vi "op_Pixel sweep.vi"(0 "EQ folder path Refnum":refnum<vi>, 1 "HV enable button":bool caption="High Voltage enable", 2 "HV parameters Refnum":refnum<vi>, 3 "HV level Refnum":refnum<vi>, 4 "HV string Refnum":refnum<vi>, 5 "Stop ACQ button Refnum":refnum<vi>, 6 "ACQ Parameters (cluster)":T2={"Acquisition Mode"=0, "Pulse width"=0, "DTP period"=1, "Number of events"=4000} caption="Acquisition Parameters" {"Number of events" min=1; "DTP period" min=1; "Pulse width" items=["25 ns", "50 ns", "75 ns", "100 ns"]; "Acquisition Mode" items=["Normal", "Pedestal", "Test Pulse", "Test Pulse trigger & synchronous"]}, 7 "Events to acquire Refnum":refnum<vi>, 8 "error tick Refnum":refnum<vi>, 9 "ACQ events fets Refnum":refnum<vi>, 10 "Operation text Refnum":refnum<vi>, 11 "ACQ events fets A Refnum":refnum<vi>, 12 "Busy Refnum":refnum<vi>, 13 "ACQ events fets B Refnum":refnum<vi>, 14 "Addresses Cluster":T1={"ENA1"=FALSE, "IP address 1"="172.16.14.22", "ENA2"=FALSE, "IP address 2"="172.16.14.23"}, 15 "etapa# terminals refnums":T3, 17 "GbReg params":u8[](array[numeric])=[32, 32], 19 "LayerChipIDs":u16[](array[numeric])=[65535, 65535] format="%04x", 27 "Itest parameter":cluster{"Itest tipus":bool, "I test":u8}={"Itest tipus"=TRUE, "I test"=1} caption="I test parameter" {"I test" max=63 step=1}) -> (23 "Folder path: acquisition reports":path=path "C:/VIPauto/Files/LayerID/Acquisition/yyyymmdd_hh-mm-ss_Leak#_HV#")   [LabVIEW 2015, in "VIPM2.lvlib"]
uses:
  VIPM2.lvlib
panel:
  out "Chip ID list 2":u32[](array[numeric]) format="%.0x"
  out "Layer ID list 2 (ordered)":u32[](array[numeric]) format="%.0x"
  out "All ID list 2":u32[](array[numeric]) format="%.0x"
  out "All ID list 1":u32[](array[numeric]) format="%.0x"
  out "Layer ID list 1 (ordered)":u32[](array[numeric]) format="%.0x"
  out "Chip ID list 1":u32[](array[numeric]) format="%.0x"
  # "Operation: Pixel sweep ACQuisition, with HV (refnums)"
  # "Analog Vref low"
  # "Gb THLD"
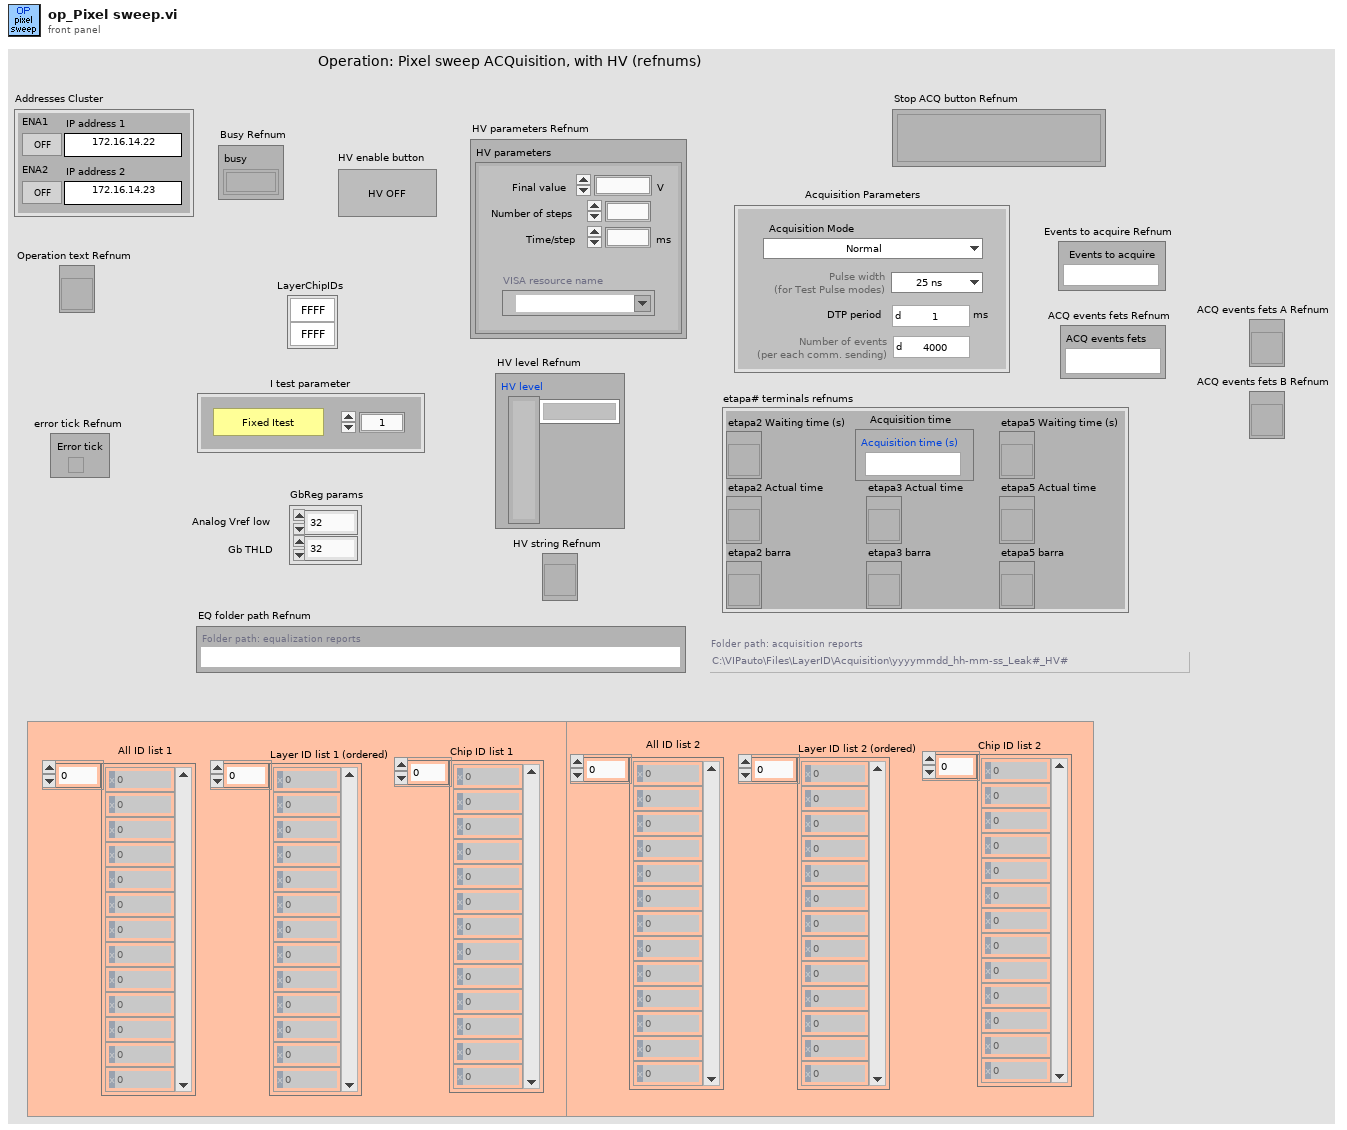
[diagram p1: front panel]
types:
  T1 = cluster{"ENA1":bool, "IP address 1":string, "ENA2":bool, "IP address 2":string}
  T2 = cluster{"Acquisition Mode":u32, "Pulse width":u32, "DTP period":u32, "Number of events":u32}
  T3 = cluster{"etapa2 Waiting time (s)":refnum<vi>, "etapa2 Actual time":refnum<vi>, "etapa2 barra":refnum<vi>, "etapa3 Actual time":refnum<vi>, "etapa3 barra":refnum<vi>, "etapa5 Waiting time (s)":refnum<vi>, "etapa5 Actual time":refnum<vi>, "etapa5 barra":refnum<vi>, "Acquisition time":refnum<vi>}
  T4 = enum8{"Enabled", "Disabled", "Disabled and Grayed Out"}
  T5 = cluster{"Final value":i16, "Number of steps":u8, "Time/step":u16, "Output Off Behavior":u16, "VISA resource name":refnum<visa-resource-name>}
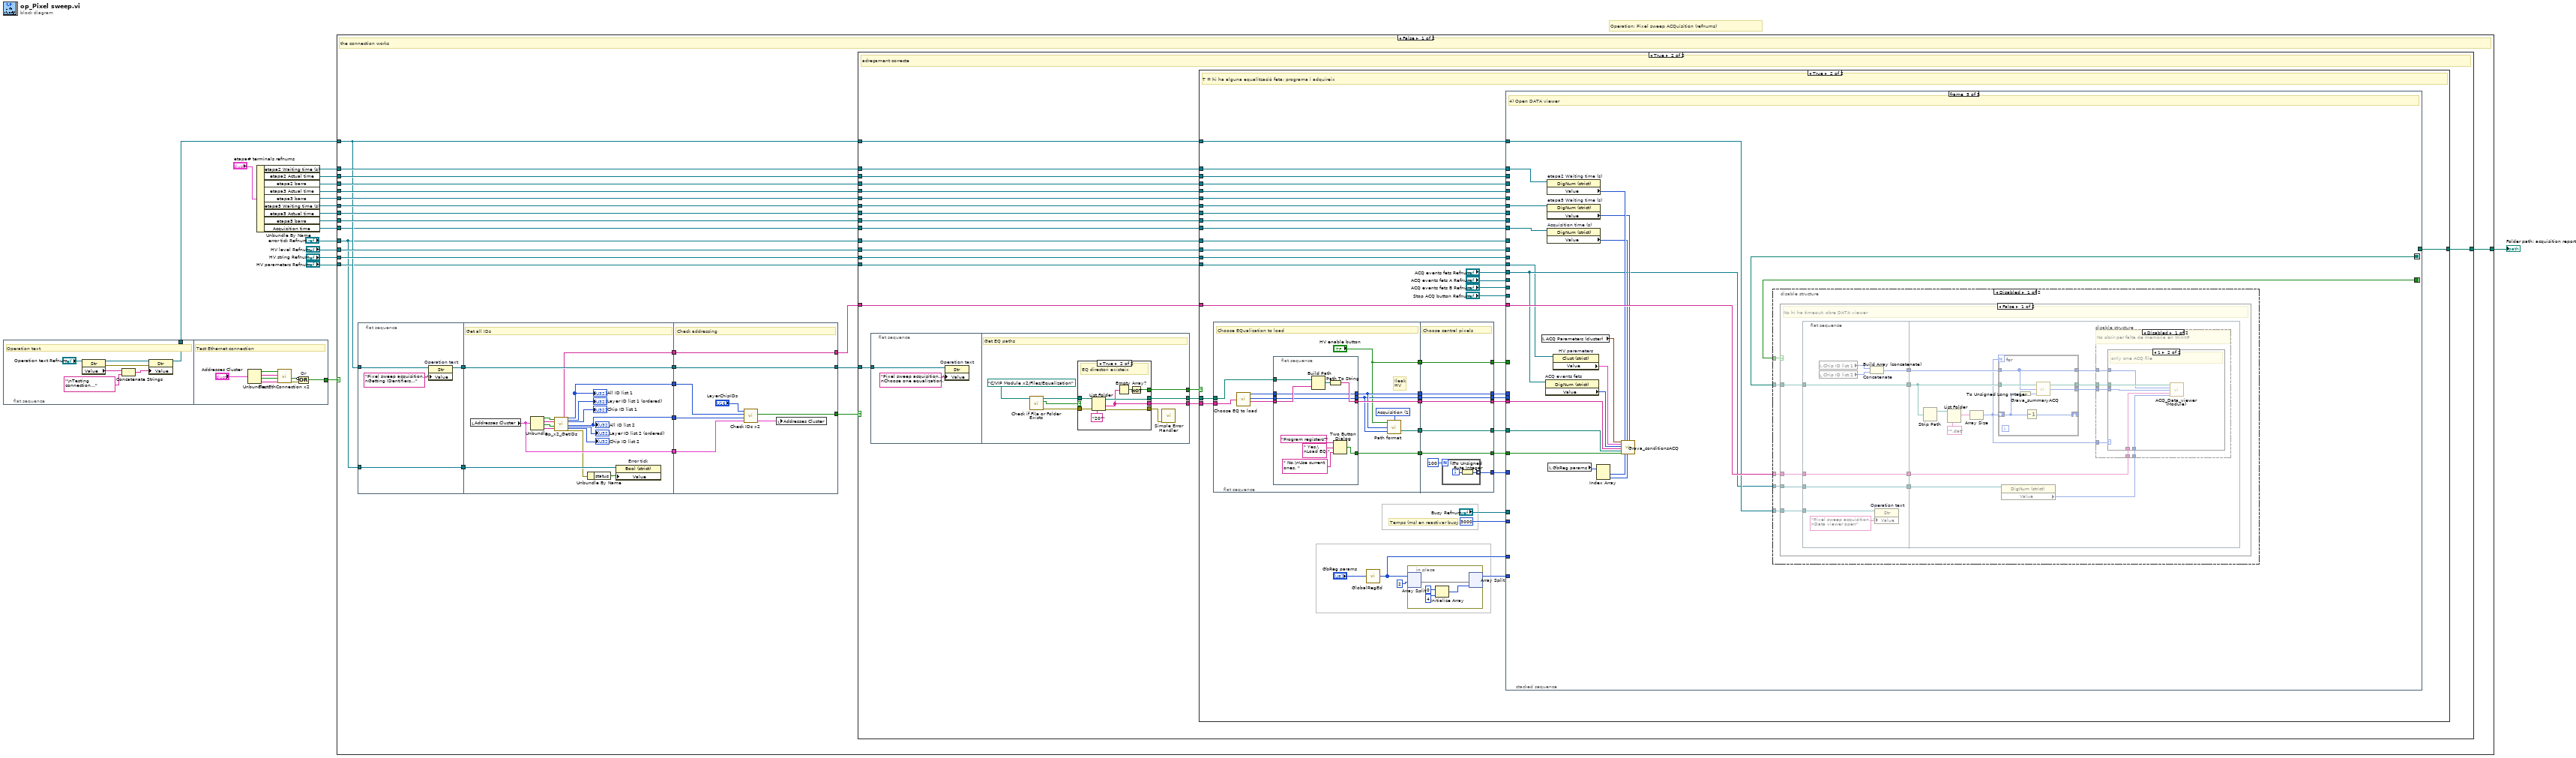
[diagram p0: block diagram]
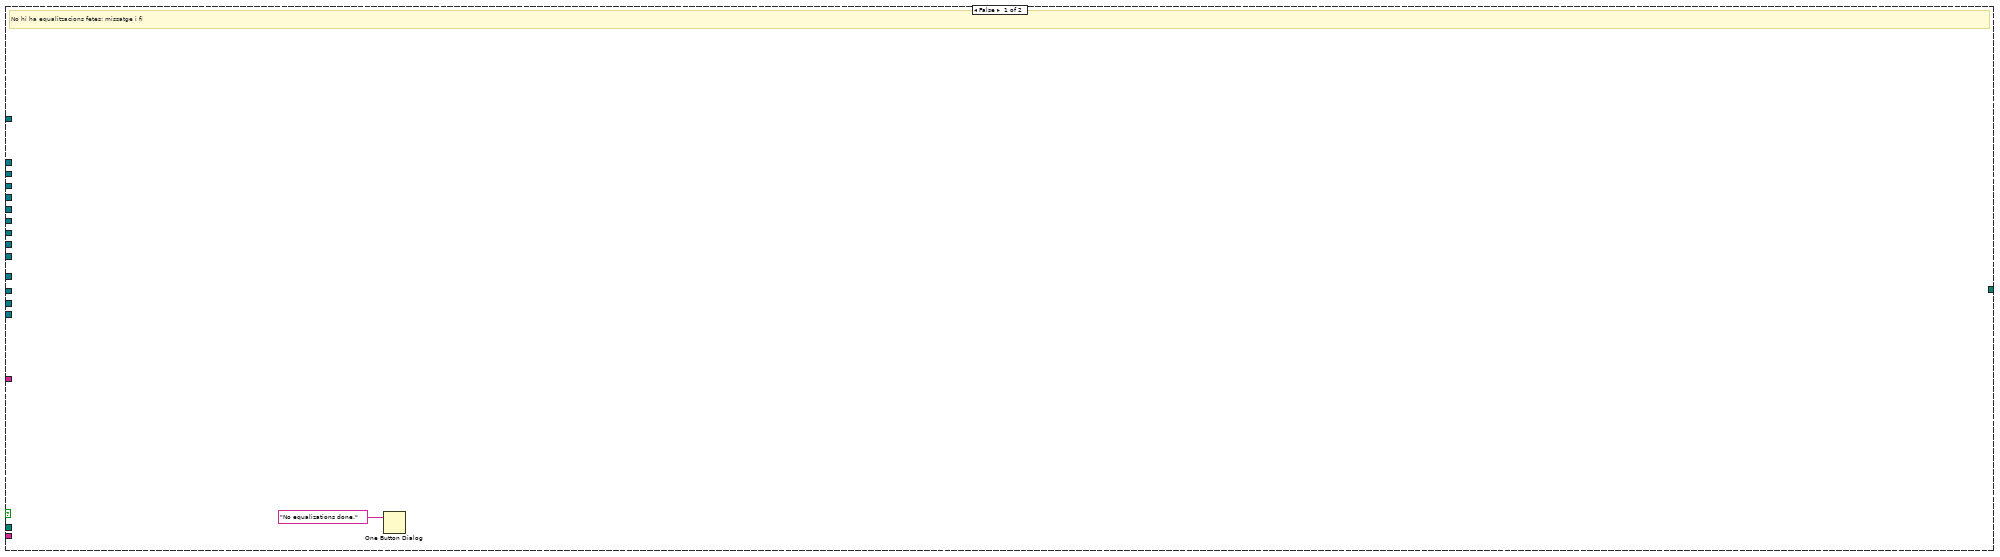
[diagram p4: hidden frame]
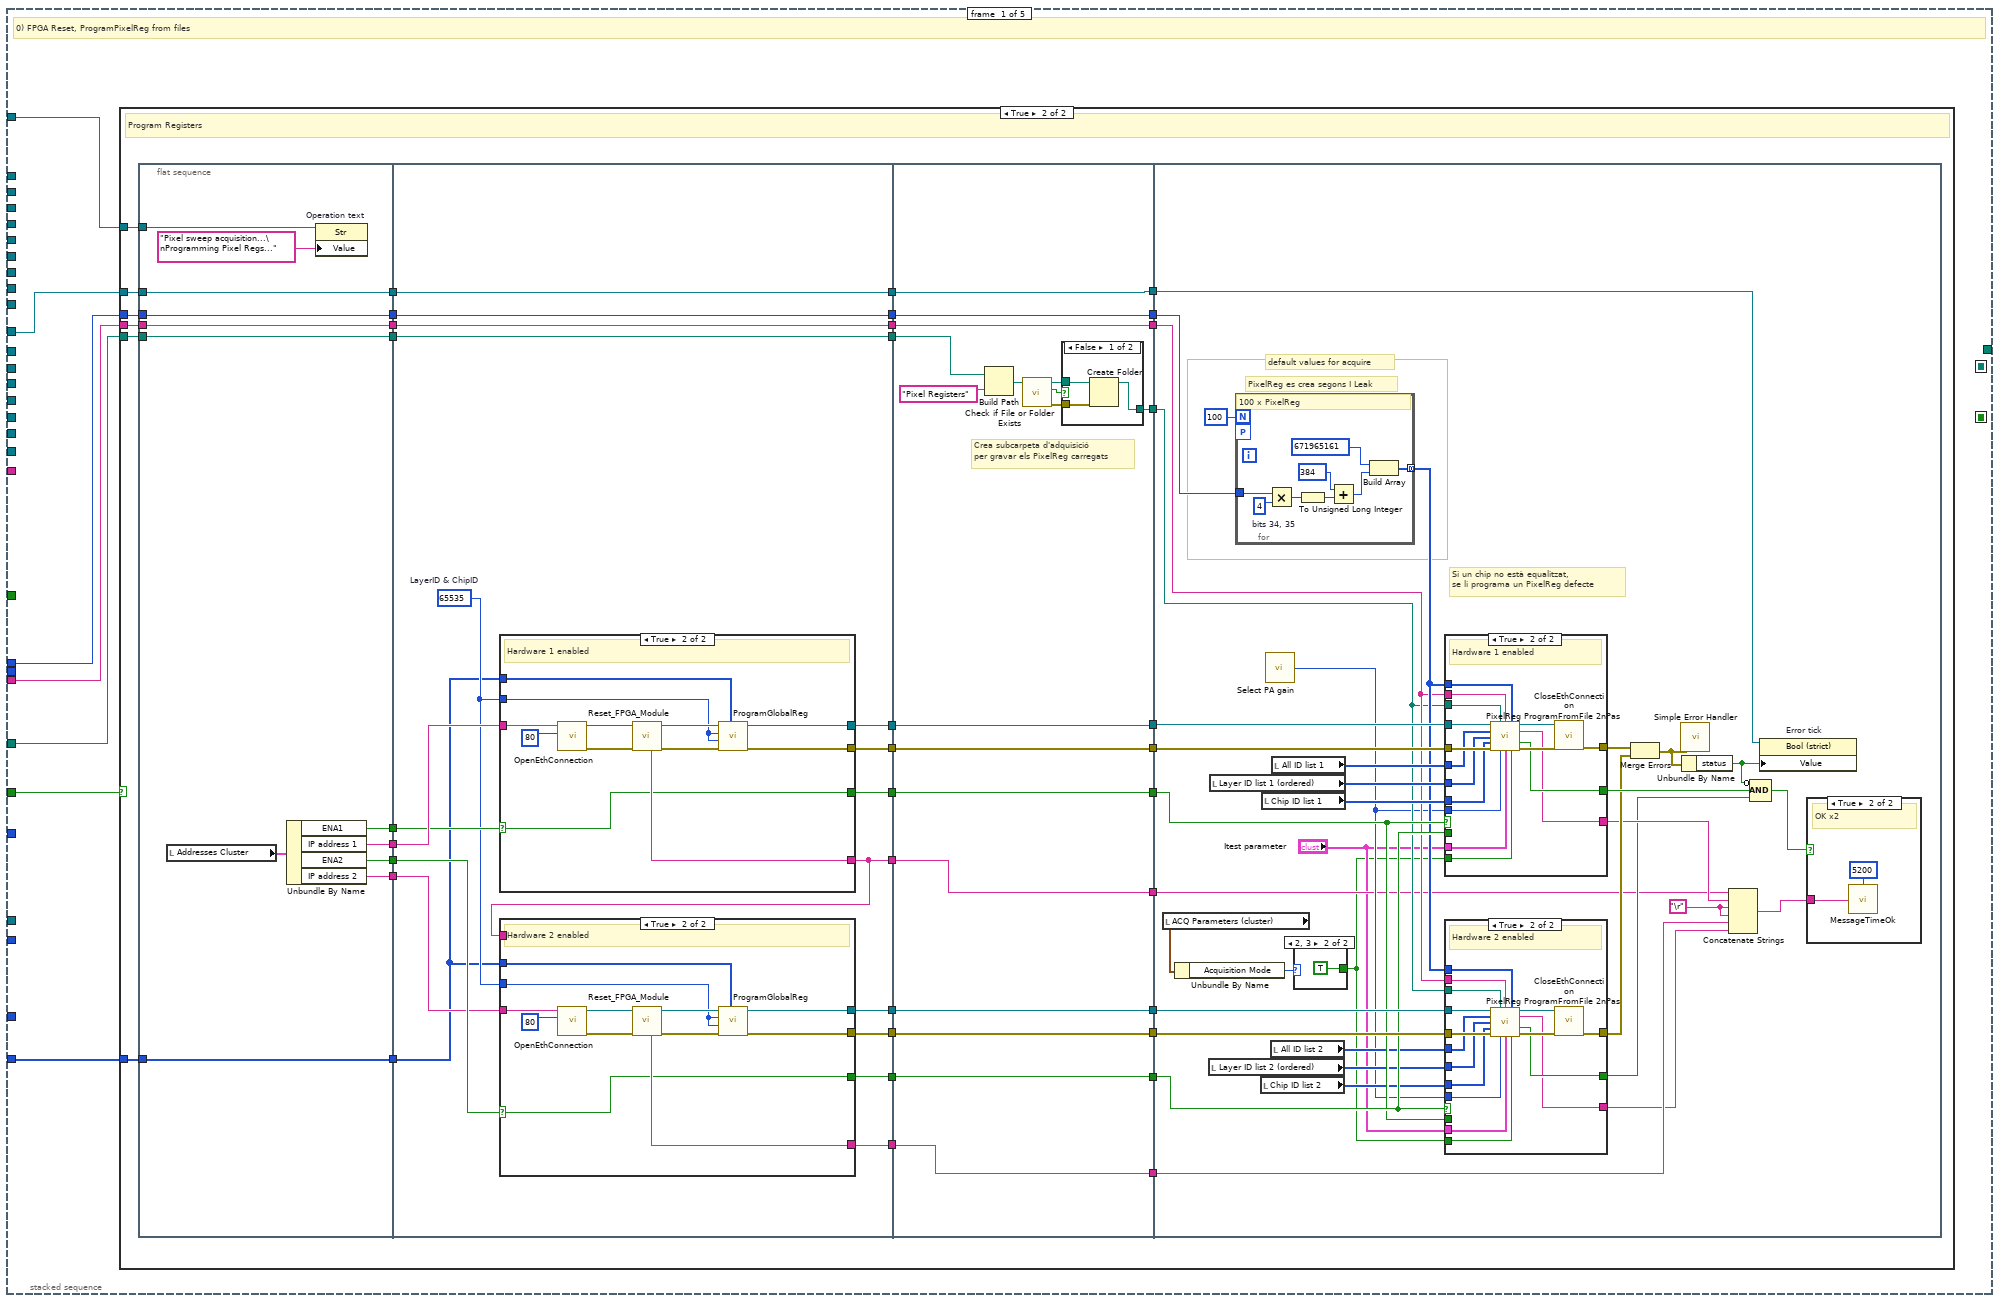
[diagram p5: hidden frame]
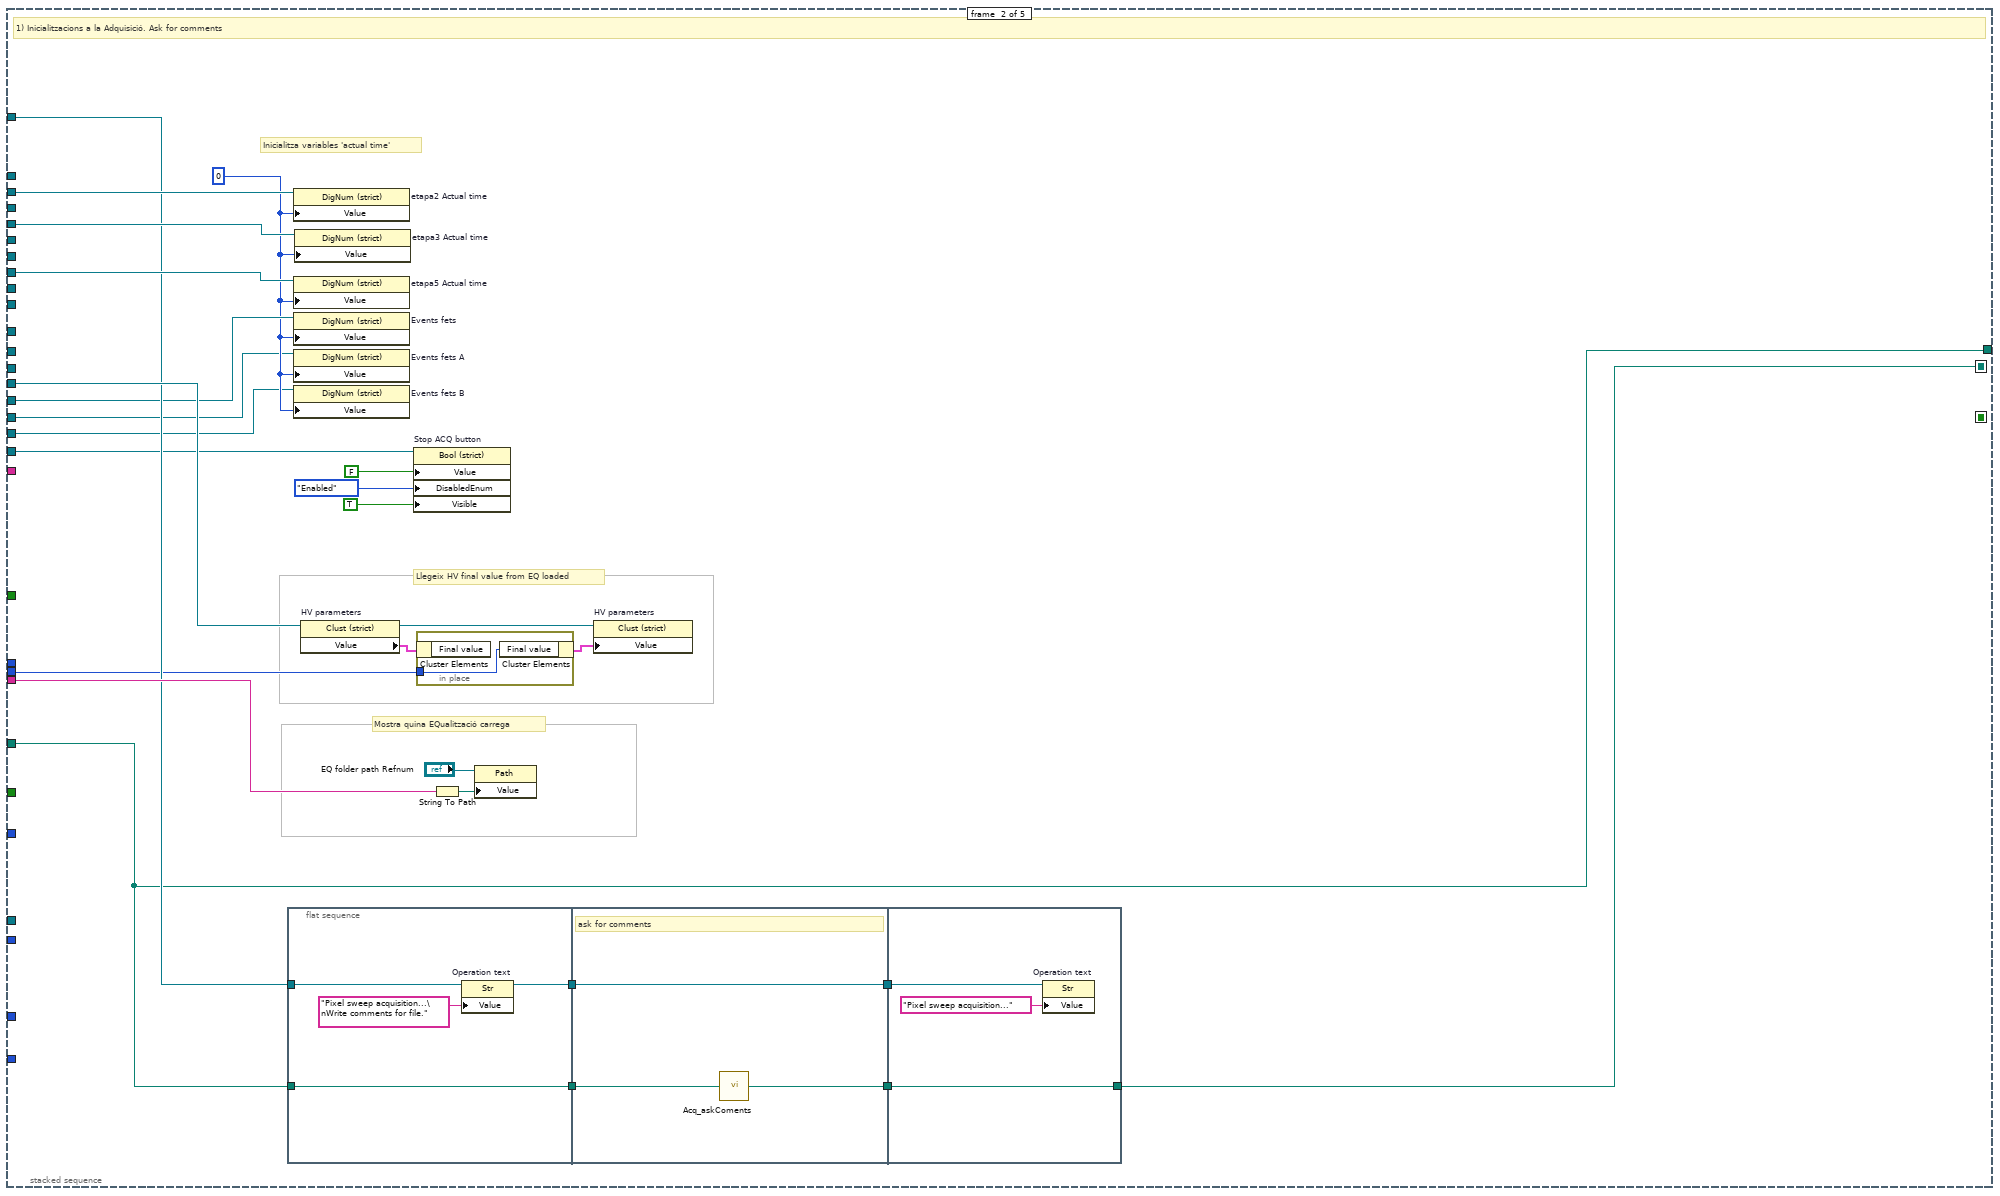
[diagram p14: hidden frame]
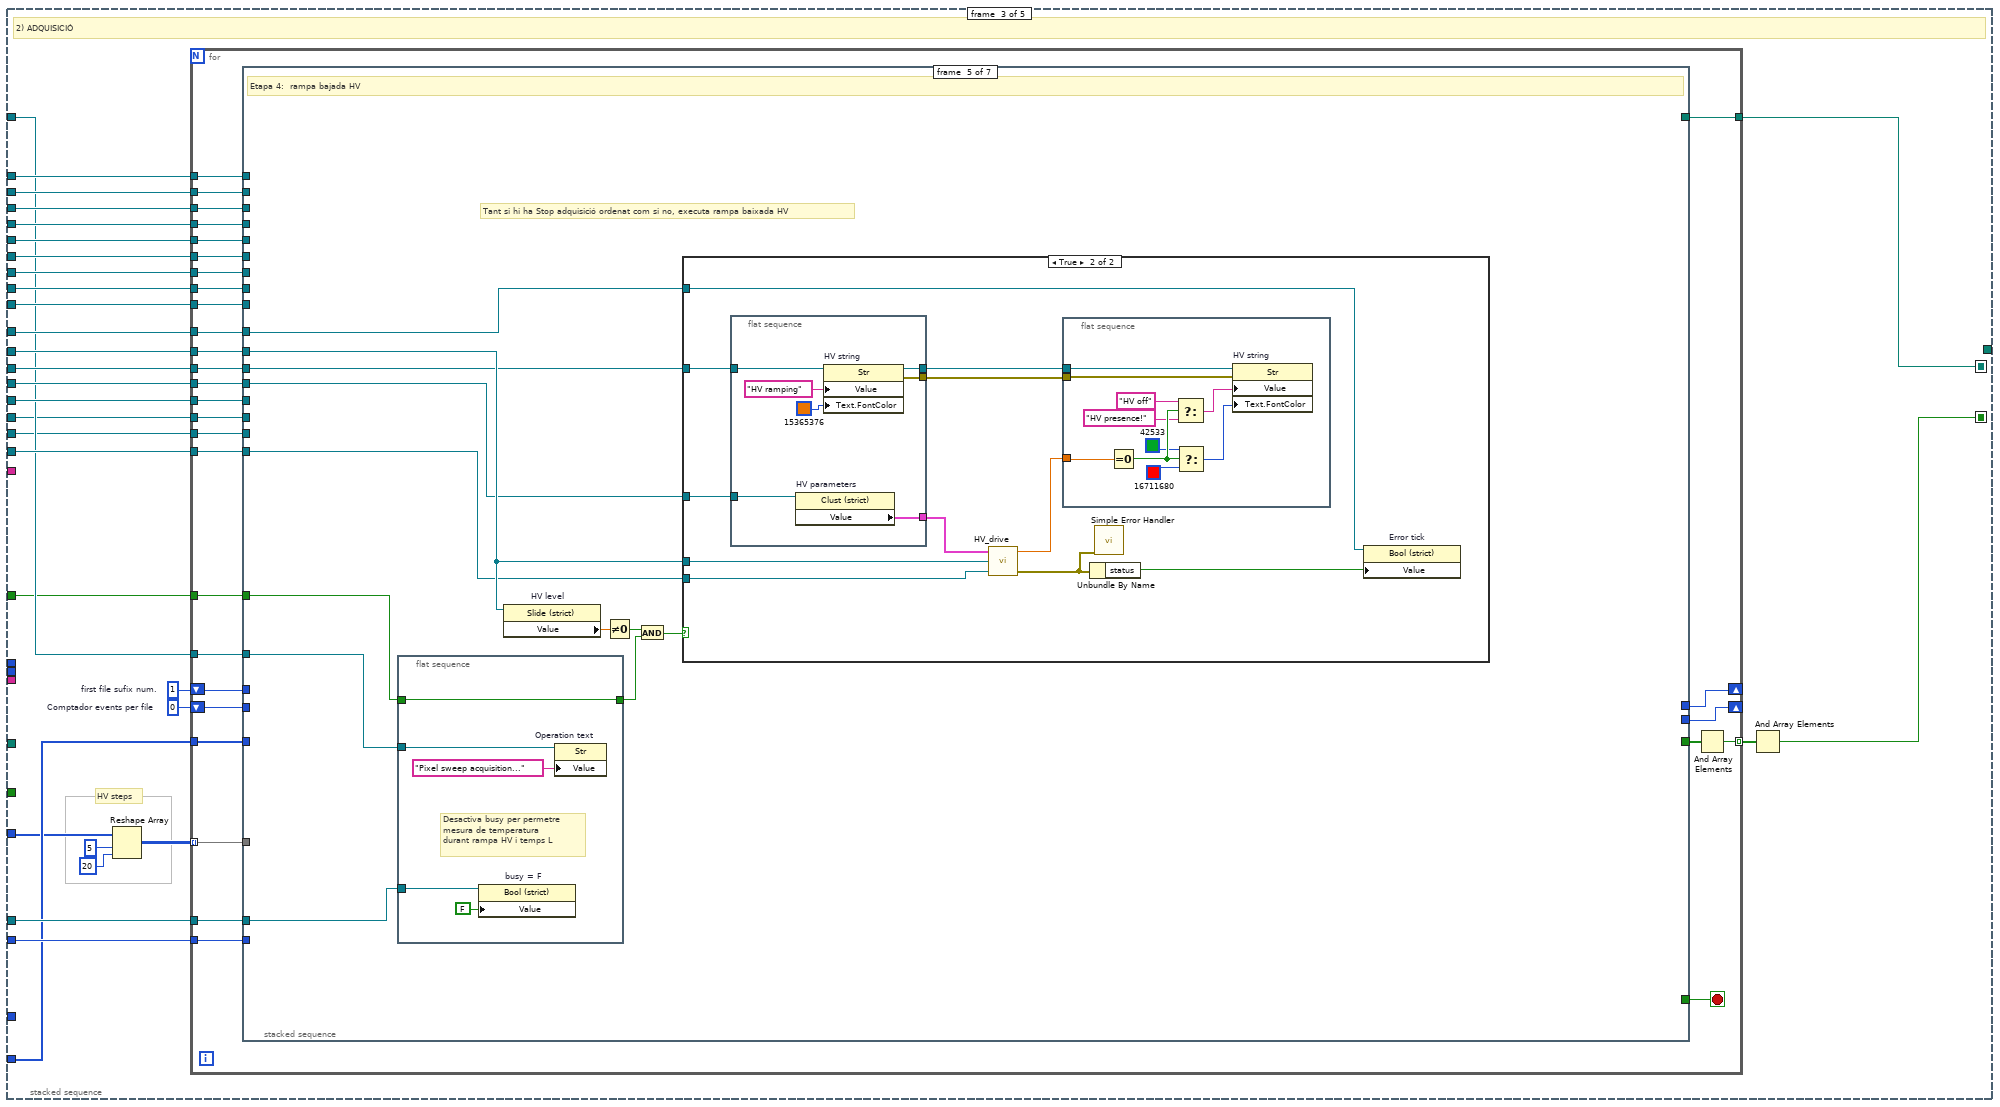
[diagram p15: hidden frame]
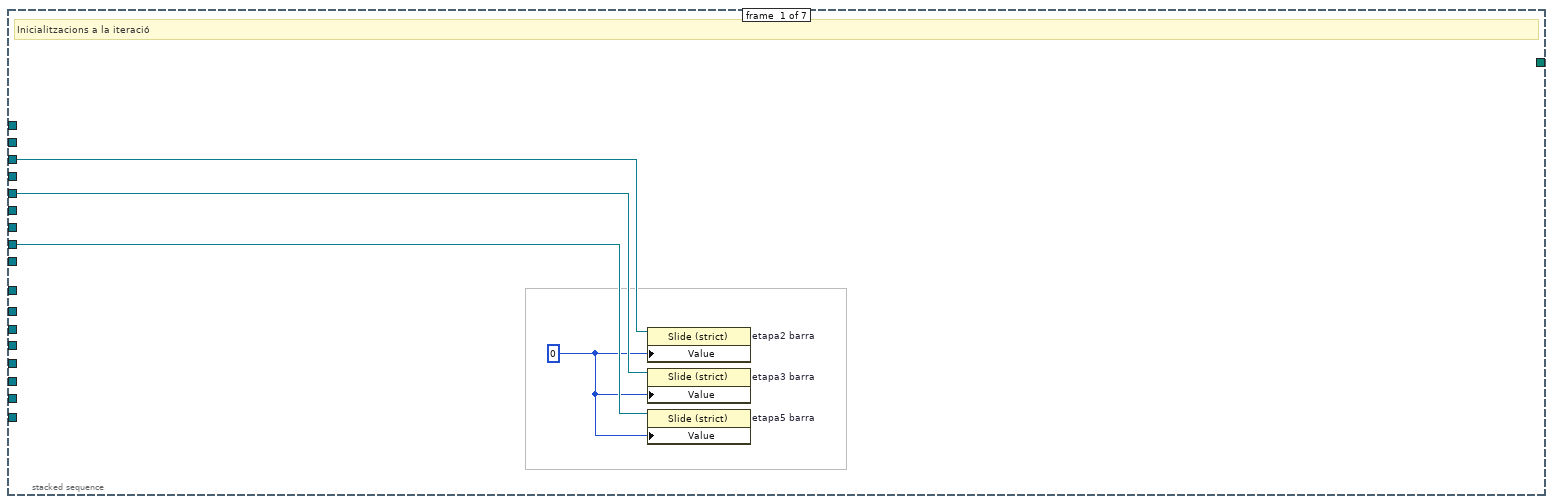
[diagram p16: hidden frame]
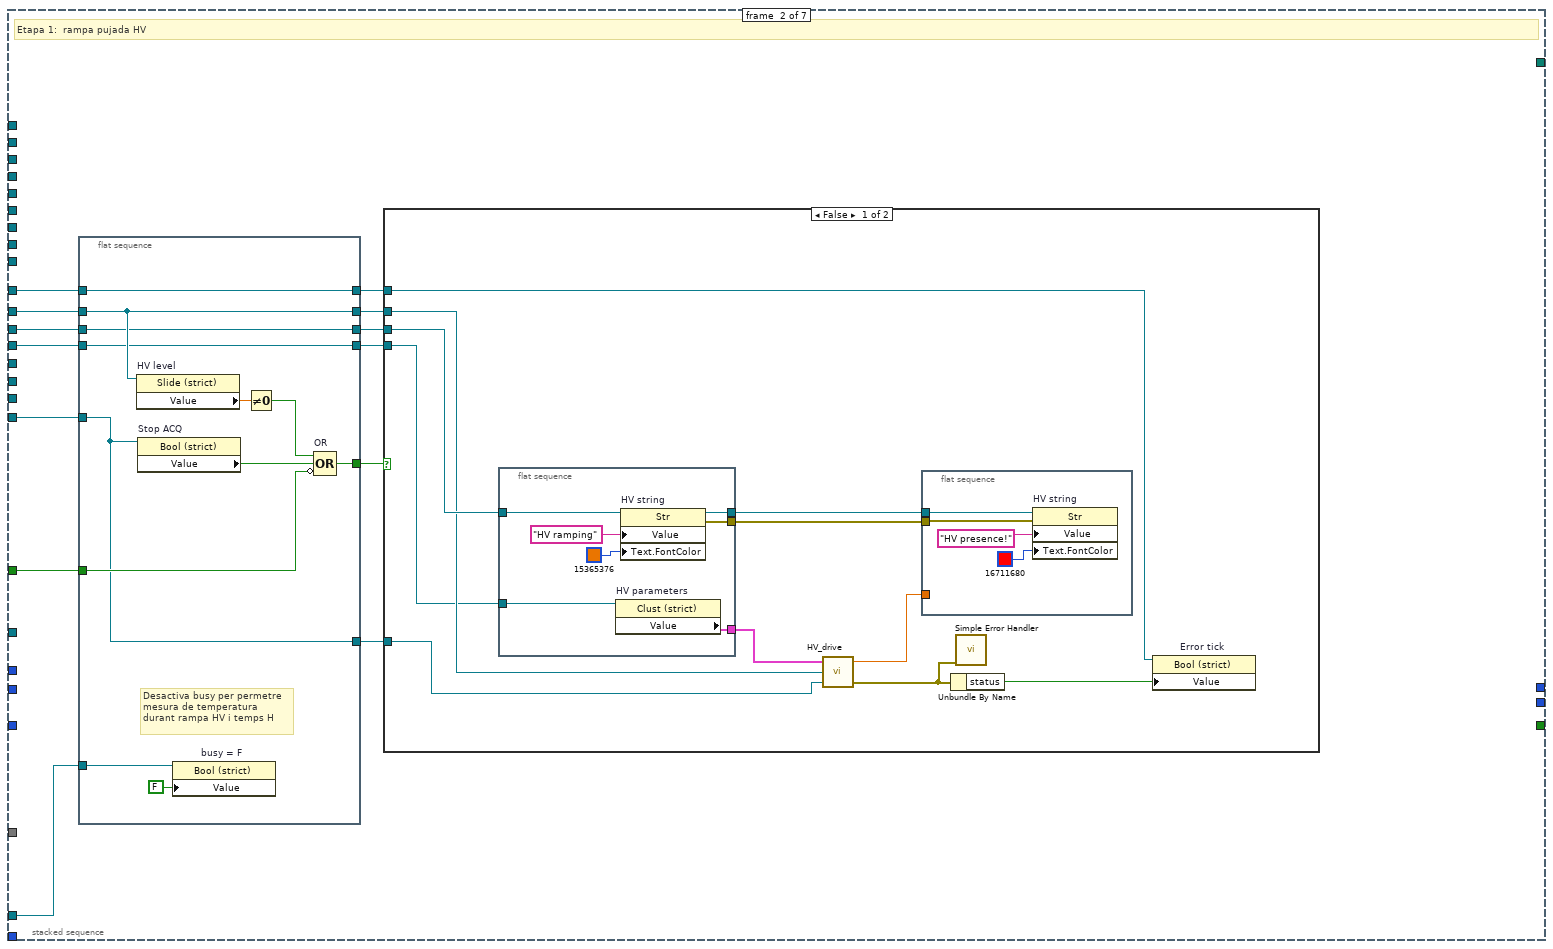
[diagram p17: hidden frame]
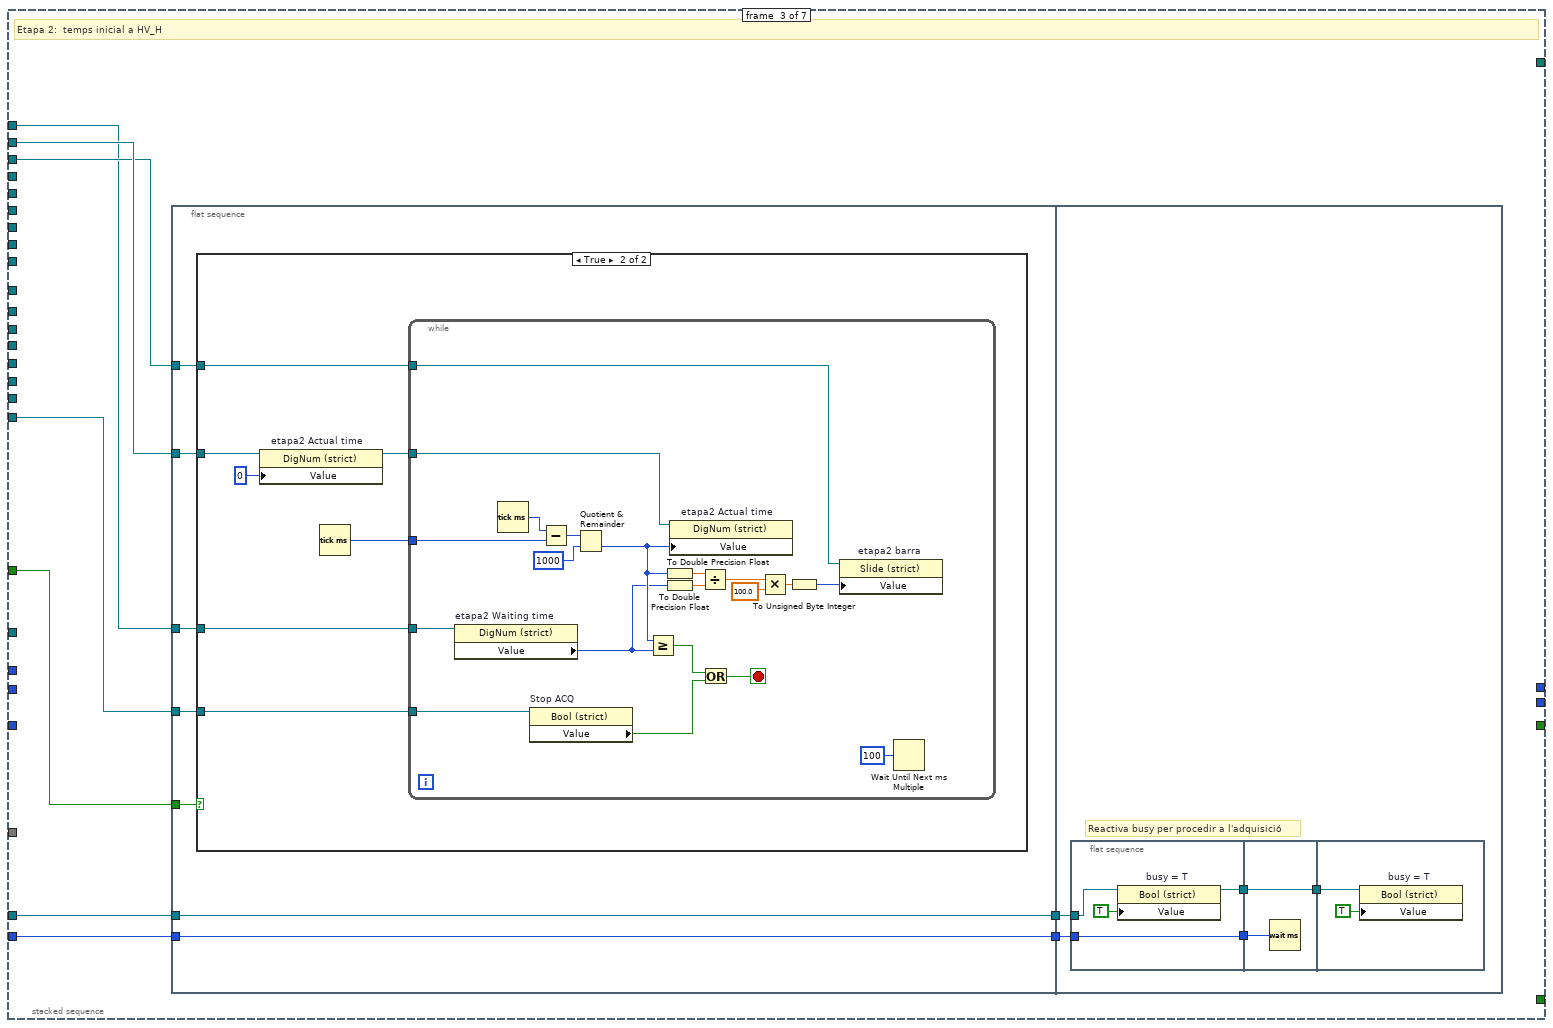
[diagram p19: hidden frame]
diagram:
  # "Operation: Pixel sweep ACQuisition (refnums)"
  n1 = flat-sequence {
    tunnel: [w18] -> w7
    tunnel: [w30] -> w17
    frame #0 {
      # "Operation text"
      n2 = property class="Str"(reference="Operation text Refnum") -> (reference out=w21:refnum<vi>, error out=w20:errorcluster, "Value"=w23:string)  [unwired: 1 in]
      n3 = Concatenate Strings "Concatenate Strings"(w23, "\nTesting connection..." ("string")) -> (w19:string)
      n4 = property class="Str"(reference=w21, error in=w20, "Value"=w19) -> (reference out=w18:refnum<vi>)  [unwired: 1 out]
    }
    frame #1 {
      # "Test Ethernet connection"
      n5 = Unbundle("Addresses Cluster") -> ("ENA1"=w28:bool, "IP address 1"=w27:string, "ENA2"=w26:bool, "IP address 2"=w25:string)
      n6 = call "TestEthConnection x2.vi"("IP address 2"=w25, "ENA2"=w26, "IP address 1"=w27, "ENA1"=w28) -> ("error out"=w31:errorcluster, "Answers OK?"=w32:bool)  [unwired: 6 in]
      n7 = Compound Arithmetic op=OR "Or"(invert w32, w31) -> (w30:bool)
    }
  }
  n8 = Unbundle By Name("etapa# terminals refnums") -> ("etapa2 Waiting time (s)"=w15:refnum<vi>, "etapa2 Actual time"=w14:refnum<vi>, "etapa2 barra"=w13:refnum<vi>, "etapa3 Actual time"=w12:refnum<vi>, "etapa3 barra"=w11:refnum<vi>, "etapa5 Waiting time (s)"=w10:refnum<vi>, "etapa5 Actual time"=w9:refnum<vi>, "etapa5 barra"=w8:refnum<vi>, "Acquisition time"=w2:refnum<vi>)
  n9 = case shown="False" w17 {
    selector: w17 -> [_ w1034]
    tunnel: w15 -> [w57 _]
    tunnel: w14 -> [w56 _]
    tunnel: w13 -> [w55 _]
    tunnel: w12 -> [w54 _]
    tunnel: w11 -> [w53 _]
    tunnel: w10 -> [w52 _]
    tunnel: w9 -> [w51 _]
    tunnel: w8 -> [w50 _]
    tunnel: w7 -> [w46 _]
    tunnel: "HV level Refnum" -> [w49 _]
    tunnel: "HV string Refnum" -> [w48 _]
    tunnel: "error tick Refnum" -> [w43 w1033]
    tunnel: [w47 _] -> w1
    tunnel: "HV parameters Refnum" -> [w45 _]
    tunnel: w2 -> [w44 _]
    frame False {
      # "the connection works"
      n10 = flat-sequence {
        tunnel: w46 -> [w61]
        tunnel: w43 -> [w58]
        tunnel: [w60] -> w42
        tunnel: [w58] -> w41
        tunnel: w42 -> [w67]
        tunnel: w41 -> [w68]
        tunnel: [w67] -> w39
        tunnel: [w66] -> w38
        tunnel: [w65] -> w36
        tunnel: [w64] -> w35
        tunnel: [w63] -> w34
        tunnel: [w84] -> w37
        tunnel: [w85] -> w40
        tunnel: w39 -> [w85]
        tunnel: w38 -> [w84]
        tunnel: w36 -> [w81]
        tunnel: w35 -> [w82]
        tunnel: w34 -> [w83]
        tunnel: [w78] -> w33
        frame #0 {
          n11 = property on="Operation text" class="Str"(reference=w61, "Value"="Pixel sweep acquisition...\nGetting IDentifiers...") -> (reference out=w60:refnum<vi>)  [unwired: 1 in, 1 out]
        }
        frame #1 {
          # "Get all IDs"
          n12 = local read "Addresses Cluster"() -> (w63:T1)
          n13 = Unbundle(w63) -> ("ENA1"=w70:bool, "IP address 1"=w71:string, "ENA2"=w73:bool, "IP address 2"=w72:string)
          n14 = call "op_x2_GetIDs.vi"("ENA1"=w70, "IP address 1"=w71, "ENA2"=w73, "IP address 2"=w72) -> ("summary IDs"=w66:string, "All ID list 1"=w65:u32[], "Layer ID list 1 (ordered)"=→"Layer ID list 1 (ordered)":u32[], "Chip ID list 1"=→"Chip ID list 1":u32[], "All ID list 2"=w64:u32[], "Layer ID list 2 (ordered)"=→"Layer ID list 2 (ordered)":u32[], "Chip ID list 2"=→"Chip ID list 2":u32[], "error out"=w62:errorcluster)  [unwired: 16 in]
          "All ID list 1" <- w65
          "All ID list 2" <- w64
          n15 = Unbundle By Name(w62) -> ("status"=w69:bool)
          n16 = property on="Error tick" class="Bool (strict)"(reference=w68, "Value"=w69) -> ()  [unwired: 1 in, 2 out]
        }
        frame #2 {
          # "Check addressing"
          n17 = call "Check IDs x2.vi"("Addresses Cluster in"=w83, "All ID list 2"=w82, "All ID list 1"=w81, "LayerChipIDs"="LayerChipIDs") -> ("Addresses Cluster out"=w79:T1, "OK?"=w78:bool)  [unwired: 6 in]
          n18 = local write "Addresses Cluster"(w79) -> ()
        }
      }
      n19 = case shown="True" w33 {
        tunnel: w57 -> [_ w105]
        tunnel: w56 -> [_ w104]
        tunnel: w55 -> [_ w103]
        tunnel: w54 -> [_ w102]
        tunnel: w53 -> [_ w101]
        tunnel: w52 -> [_ w100]
        tunnel: w51 -> [_ w99]
        tunnel: w50 -> [_ w98]
        tunnel: w49 -> [_ w97]
        tunnel: w48 -> [_ w96]
        tunnel: [_ w95] -> w47
        tunnel: w46 -> [_ w94]
        tunnel: w45 -> [_ w90]
        tunnel: w44 -> [_ w89]
        tunnel: w43 -> [_ w88]
        tunnel: w40 -> [_ w87]
        tunnel: w37 -> [_ w86]
        frame False {
          # "adreçament incorrecte"
        }
        frame True {
          # "adreçament correcte"
          n20 = flat-sequence {
            tunnel: w87 -> [w106]
            tunnel: [w115] -> w93
            tunnel: [w114] -> w92
            tunnel: [w113] -> w91
            frame #0 {
              n21 = property on="Operation text" class="Str"(reference=w106, "Value"="Pixel sweep acquisition...\nChoose one equalization.") -> ()  [unwired: 1 in, 2 out]
            }
            frame #1 {
              # "Get EQ paths"
              n22 = call <vilib>:"Check if File or Folder Exists.vi"("path"=path "C:/VIP Module x2/Files/Equalization") -> ("error out"=w109:errorcluster, "file or folder exists?"=w110:bool, "dup path"=w111:path)  [unwired: 8 in]
              n23 = case shown="True" w110 {
                selector: w110 -> [w118 _]
                tunnel: w111 -> [w117 w124]
                tunnel: w109 -> [w116 w123]
                tunnel: [w118 w120] -> w115
                tunnel: [w117 w121] -> w114
                tunnel: [w116 w122] -> w108
                tunnel: [_ w119] -> w113
                frame False {
                  # "no EQs"
                }
                frame True {
                  # "EQ directori existeix"
                  n24 = List Folder(path=w124, pattern="20*", error in=w123) -> (path out=w121:path, folder names=w119:string[], error out=w122:errorcluster)  [unwired: 1 in, 1 out]
                  n25 = Empty Array?(array=w119) -> (empty?=w125:bool)
                  n26 = Not(x=w125) -> (.not. x?=w120:bool)
                }
              }
              n27 = call <vilib>:"Simple Error Handler.vi"("error in (no error)"=w108) -> ()  [unwired: 4 in, 5 out]
            }
          }
          n28 = case shown="True" w93 {
            tunnel: w105 -> [_ w168]
            tunnel: w104 -> [_ w167]
            tunnel: w103 -> [_ w166]
            tunnel: w102 -> [_ w165]
            tunnel: w101 -> [_ w164]
            tunnel: w100 -> [_ w163]
            tunnel: w99 -> [_ w162]
            tunnel: w98 -> [_ w161]
            tunnel: w97 -> [_ w160]
            tunnel: w96 -> [_ w159]
            tunnel: [_ w158] -> w95
            tunnel: w94 -> [_ w157]
            tunnel: w88 -> [_ w156]
            tunnel: w92 -> [_ w155]
            tunnel: w91 -> [_ w154]
            tunnel: w90 -> [_ w150]
            tunnel: w89 -> [_ w147]
            tunnel: w86 -> [_ w145]
            frame False {
              # "No hi ha equalitzacions fetes: missatge i fi"
              n29 = One Button Dialog(message="No equalizations done.") -> ()  [unwired: 1 in, 1 out]
            }
            frame True {
              # "Temps (ms) en reactivar busy"
              # "T = hi ha alguna equalització feta: programa i adquireix"
              n30 = flat-sequence {
                tunnel: w155 -> [w181]
                tunnel: w154 -> [w182]
                tunnel: [w179] -> w140
                tunnel: [w174] -> w139
                tunnel: [w177] -> w138
                tunnel: [w183] -> w137
                tunnel: [w178] -> w136
                tunnel: ["HV enable button"] -> w135
                tunnel: [w197] -> w141
                tunnel: [w198] -> w144
                tunnel: [w199] -> w149
                tunnel: [w200] -> w151
                tunnel: [w201] -> w152
                tunnel: [w202] -> w153
                tunnel: w140 -> [w202]
                tunnel: w139 -> [w201]
                tunnel: w138 -> [w200]
                tunnel: w137 -> [w199]
                tunnel: w136 -> [w198]
                tunnel: w135 -> [w197]
                tunnel: [w195] -> w134
                frame #0 {
                  w184 = u8 1 items=["Equalization", "Acquisition"] ("Operation type")
                  # "Ileak\nHV"
                  # "Choose EQualization to load"
                  n31 = call "Choose EQ to load.vi"("EQ folders"=w182) -> ("I Leakage"=w176:u8, "HV last value"=w175:i16, "loaded EQ folder"=w180:string)  [unwired: 5 in]
                  n32 = flat-sequence {
                    tunnel: w181 -> [w194]
                    tunnel: w180 -> [w193]
                    tunnel: [w191] -> w179
                    tunnel: [w190] -> w178
                    tunnel: [w186] -> w177
                    tunnel: w176 -> [w186]
                    tunnel: w175 -> [w185]
                    tunnel: [w185] -> w174
                    frame #0 {
                      n33 = Build Path(base path=w194, name or relative path=w193) -> (appended path=w192:path)
                      n34 = Path To String(path=w192) -> (string=w191:string)
                      n35 = Two Button Dialog(message="Program registers?", 1:" No.\nUse current ones. " ("F button name (\"Cancel\")"), 2:" Yes.\nLoad EQ." ("T button name (\"OK\")")) -> (T button?=w190:bool)
                    }
                  }
                  n36 = call "Path format.vi"("Operation type"=w184, "HV level"=w174, "I leakage"=w177, "HV enable button"="HV enable button") -> ("folder path"=w183:path)  [unwired: 1 in]
                }
                frame #1 {
                  # "Choose central pixels"
                  n37 = for {
                    N: 100 -> [_]
                    tunnel: [w203] -> w195 mode=indexing
                    i -> [w204]
                    n38 = To Unsigned Byte Integer(number=w204) -> (unsigned 8bit integer=w203:u8)
                  }
                }
              }
              n39 = call "GlobalRegEd.vi"("params"="GbReg params") -> ("Global Reg out"=w129:u32[])  [unwired: 4 in]
              n40 = in-place {
                n41 = in-place-split #1(w129, 2) -> (w172:u32[])  [unwired: 1 out]
                n42 = Initialize Array "Initialize Array"(u32 0, 4 ("dimension size")) -> (w169:u32[])
                n43 = in-place-split #1(w172, w169) -> (w130:u32[])  [unwired: 1 out]
              }
              n44 = stacked-sequence {
                seq-local: [_ _ w449 _ _] -> [_ _ _ _ w979]
                seq-local: [_ w422 _ _ _] -> [_ _ w465 _ w978]
                tunnel: w157 -> [w211 w427 w461 w899 w976]
                tunnel: w168 -> [_ _ w479 _ w959]
                tunnel: w167 -> [_ w437 w478 _ _]
                tunnel: w166 -> [_ _ w477 _ _]
                tunnel: w165 -> [_ w436 w476 _ _]
                tunnel: w164 -> [_ _ w475 _ _]
                tunnel: w163 -> [_ _ w474 _ w960]
                tunnel: w162 -> [_ w435 w473 _ _]
                tunnel: w161 -> [_ _ w472 _ _]
                tunnel: w156 -> [w210 _ w469 w901 _]
                tunnel: w160 -> [_ _ w471 _ _]
                tunnel: w159 -> [_ _ w470 _ _]
                tunnel: [_ w420 _ _ _] -> w158
                tunnel: w153 -> [w209 w428 _ _ w964]
                tunnel: w152 -> [_ w426 _ _ _]
                tunnel: w151 -> [w208 _ _ _ _]
                tunnel: w150 -> [_ w434 w468 _ w962]
                tunnel: w149 -> [w207 w420 _ _ w965]
                tunnel: "Stop ACQ button Refnum" -> [_ w419 w467 w898 _]
                tunnel: w147 -> [_ _ w466 _ w961]
                tunnel: "ACQ events fets Refnum" -> [_ w415 w464 _ w963]
                tunnel: w145 -> [_ _ _ _ w977]
                tunnel: w144 -> [w206 _ _ _ w966]
                tunnel: "Busy Refnum" -> [_ _ w463 w897 _]
                tunnel: u32 3000 -> [_ _ w462 _ _]
                tunnel: w141 -> [_ _ w460 _ _]
                tunnel: w134 -> [_ _ w454 _ _]
                tunnel: "ACQ events fets A Refnum" -> [_ w413 w459 _ _]
                tunnel: "ACQ events fets B Refnum" -> [_ w412 w458 _ _]
                tunnel: w130 -> [w205 _ w455 _ _]
                tunnel: w129 -> [_ _ _ w896 _]
                frame #0 {
                  # "0) FPGA Reset, ProgramPixelReg from files"
                  n45 = case shown="True" w206 {
                    tunnel: w211 -> [_ w237]
                    tunnel: w210 -> [_ w236]
                    tunnel: w209 -> [_ w235]
                    tunnel: w208 -> [_ w234]
                    tunnel: w207 -> [_ w233]
                    tunnel: w205 -> [_ w213]
                    frame False {
                      # "Use current registers values"
                    }
                    frame True {
                      # "Program Registers"
                      n46 = flat-sequence {
                        tunnel: w237 -> [w261]
                        tunnel: [w260] -> w250
                        tunnel: w236 -> [w260]
                        tunnel: [w259] -> w249
                        tunnel: w235 -> [w259]
                        tunnel: [w258] -> w248
                        tunnel: w234 -> [w258]
                        tunnel: [w257] -> w247
                        tunnel: w233 -> [w257]
                        tunnel: [w255] -> w232
                        tunnel: [w254] -> w231
                        tunnel: [w253] -> w230
                        tunnel: [w252] -> w229
                        tunnel: w213 -> [w251]
                        tunnel: [w251] -> w212
                        tunnel: [w280] -> w246
                        tunnel: w250 -> [w280]
                        tunnel: w249 -> [w279]
                        tunnel: [w279] -> w245
                        tunnel: w248 -> [w278]
                        tunnel: [w278] -> w244
                        tunnel: w247 -> [w277]
                        tunnel: [w277] -> w243
                        tunnel: w232 -> [w272]
                        tunnel: w231 -> [w267]
                        tunnel: w230 -> [w273]
                        tunnel: w229 -> [w266]
                        tunnel: [w276] -> w228
                        tunnel: [w275] -> w227
                        tunnel: [w274] -> w226
                        tunnel: [w263] -> w225
                        tunnel: [w271] -> w224
                        tunnel: [w270] -> w223
                        tunnel: [w269] -> w222
                        tunnel: [w268] -> w221
                        tunnel: w212 -> [w264]
                        tunnel: [w314] -> w242
                        tunnel: [w313] -> w241
                        tunnel: [w324] -> w240
                        tunnel: w246 -> [w324]
                        tunnel: [w323] -> w239
                        tunnel: w245 -> [w323]
                        tunnel: [w322] -> w238
                        tunnel: w244 -> [w322]
                        tunnel: w243 -> [w316]
                        tunnel: w228 -> [w314]
                        tunnel: w227 -> [w313]
                        tunnel: w226 -> [w312]
                        tunnel: w225 -> [w308]
                        tunnel: w224 -> [w311]
                        tunnel: w223 -> [w310]
                        tunnel: w222 -> [w309]
                        tunnel: w221 -> [w307]
                        tunnel: [w315] -> w220
                        tunnel: [w312] -> w219
                        tunnel: [w311] -> w218
                        tunnel: [w310] -> w217
                        tunnel: [w309] -> w216
                        tunnel: [w308] -> w215
                        tunnel: [w307] -> w214
                        tunnel: w242 -> [w359]
                        tunnel: w241 -> [w358]
                        tunnel: w240 -> [w361]
                        tunnel: w239 -> [w341]
                        tunnel: w238 -> [w356]
                        tunnel: w220 -> [w340]
                        tunnel: w219 -> [w349]
                        tunnel: w218 -> [w352]
                        tunnel: w217 -> [w351]
                        tunnel: w216 -> [w350]
                        tunnel: w215 -> [w334]
                        tunnel: w214 -> [w337]
                        frame #0 {
                          n47 = local read "Addresses Cluster"() -> (w256:T1)
                          n48 = Unbundle By Name(w256) -> ("ENA1"=w255:bool, "IP address 1"=w253:string, "ENA2"=w254:bool, "IP address 2"=w252:string)
                          n49 = property on="Operation text" class="Str"(reference=w261, "Value"="Pixel sweep acquisition...\nProgramming Pixel Regs...") -> ()  [unwired: 1 in, 2 out]
                        }
                        frame #1 {
                          w265 = u32 65535  # LayerID & ChipID
                          n50 = case shown="True" w272 {
                            selector: w272 -> [w294 w295]
                            tunnel: w265 -> [_ w297]
                            tunnel: [_ w301] -> w276
                            tunnel: [_ w300] -> w275
                            tunnel: [_ w299] -> w263
                            tunnel: w264 -> [_ w298]
                            tunnel: w273 -> [_ w296]
                            tunnel: [w294 w295] -> w274
                            frame False {
                              # "Hardware 1 not enabled"
                            }
                            frame True {
                              # "Hardware 1 enabled"
                              n51 = call "OpenEthConnection.vi"("Port"=u16 80, "IP address"=w296) -> ("error out"=w305:errorcluster, "connection ID out"=w306:refnum<k5>)  [unwired: 7 in, 1 out]
                              n52 = call "Reset_FPGA_Module.vi"("error in (no error)"=w305, "connection ID"=w306) -> ("error out"=w302:errorcluster, "connection ID out"=w303:refnum<k5>, "Answer to Reset"=w299:string)  [unwired: 7 in]
                              n53 = call "ProgramGlobalReg.vi"("Global Reg"=w298, "error in (no error)"=w302, "ChipID"=w297, "LayerID"=w297, "connection ID"=w303) -> ("error out"=w300:errorcluster, "connection ID out"=w301:refnum<k5>)  [unwired: 2 in, 3 out]
                            }
                          }
                          n54 = case shown="True" w267 {
                            selector: w267 -> [w281 w282]
                            tunnel: w265 -> [_ w284]
                            tunnel: [_ w288] -> w271
                            tunnel: [_ w287] -> w270
                            tunnel: [_ w286] -> w268
                            tunnel: w264 -> [_ w285]
                            tunnel: w266 -> [_ w283]
                            tunnel: [w281 w282] -> w269
                            tunnel: w263 -> [_ _]
                            frame False {
                              # "Hardware 2 not enabled"
                            }
                            frame True {
                              # "Hardware 2 enabled"
                              n55 = call "OpenEthConnection.vi"("Port"=u16 80, "IP address"=w283) -> ("error out"=w292:errorcluster, "connection ID out"=w293:refnum<k5>)  [unwired: 7 in, 1 out]
                              n56 = call "Reset_FPGA_Module.vi"("error in (no error)"=w292, "connection ID"=w293) -> ("error out"=w289:errorcluster, "connection ID out"=w290:refnum<k5>, "Answer to Reset"=w286:string)  [unwired: 7 in]
                              n57 = call "ProgramGlobalReg.vi"("Global Reg"=w285, "error in (no error)"=w289, "ChipID"=w284, "LayerID"=w284, "connection ID"=w290) -> ("error out"=w287:errorcluster, "connection ID out"=w288:refnum<k5>)  [unwired: 2 in, 3 out]
                            }
                          }
                        }
                        frame #2 {
                          # "Crea subcarpeta d'adquisició\nper gravar els PixelReg carregats"
                          n58 = Build Path(base path=w316, name or relative path="Pixel Registers") -> (appended path=w320:path)
                          n59 = call <vilib>:"Check if File or Folder Exists.vi"("path"=w320) -> ("error out"=w317:errorcluster, "file or folder exists?"=w319:bool, "dup path"=w318:path)  [unwired: 8 in]
                          n60 = case shown="False" w319 {
                            tunnel: w318 -> [w327 w328]
                            tunnel: w317 -> [w326 _]
                            tunnel: [w325 w328] -> w315
                            frame False {
                              n61 = Create Folder(path (use dialog)=w327, error in=w326) -> (created path=w325:path)  [unwired: 1 in, 2 out]
                            }
                            frame True {
                            }
                          }
                        }
                        frame #3 {
                          w338 = "\r"
                          # "Si un chip no està equalitzat,\nse li programa un PixelReg defecte"
                          # "default values for acquire"
                          # "PixelReg es crea segons I Leak"
                          n62 = local read "ACQ Parameters (cluster)"() -> (w331:T2)
                          n63 = Unbundle By Name(w331) -> ("Acquisition Mode"=w330:u32)
                          n64 = local read "Layer ID list 2 (ordered)"() -> (w347:u32[])
                          n65 = local read "Layer ID list 1 (ordered)"() -> (w354:u32[])
                          n66 = for {
                            N: 100 -> [_]
                            tunnel: w356 -> [w405]
                            tunnel: [w402] -> w342 mode=concatenating
                            workers-P: _ -> [_]
                            w409 = u8 4  # bits 34, 35
                            # "100 x PixelReg"
                            n67 = Multiply(x=w405, y=w409) -> (x*y=w407:u8)
                            n68 = To Unsigned Long Integer(number=w407) -> (unsigned 32bit integer=w406:u32)
                            n69 = Add(x=u32 384, y=w406) -> (x+y=w403:u32)
                            n70 = Build Array(u32 671965161 ("Numeric"), w403) -> (w402:u32[])
                          }
                          n71 = local read "Chip ID list 2"() -> (w346:u32[])
                          n72 = local read "Chip ID list 1"() -> (w353:u32[])
                          n73 = call "Select PA gain.vi"() -> ("PA gain selected"=w336:u8)  [unwired: 5 in]
                          n74 = local read "All ID list 2"() -> (w348:u32[])
                          n75 = local read "All ID list 1"() -> (w355:u32[])
                          n76 = case shown="2, 3" w330 {
                            tunnel: [_ TRUE] -> w329
                            frame Default {
                            }
                            frame 2, 3 {
                            }
                          }
                          n77 = case shown="True" w349 {
                            tunnel: [w385 w401] -> w344
                            tunnel: w359 -> [_ w400]
                            tunnel: w358 -> [w385 w399]
                            tunnel: [w384 w396] -> w357
                            tunnel: w342 -> [_ w395]
                            tunnel: w341 -> [_ w394]
                            tunnel: w340 -> [_ w393]
                            tunnel: [_ w392] -> w339
                            tunnel: w355 -> [_ w389]
                            tunnel: w354 -> [_ w390]
                            tunnel: w353 -> [_ w391]
                            tunnel: w350 -> [w384 _]
                            tunnel: w336 -> [_ w388]
                            tunnel: "Itest parameter" -> [_ w387]
                            tunnel: w329 -> [_ w386]
                            frame False {
                              # "Hardware 1 not enabled"
                            }
                            frame True {
                              # "Hardware 1 enabled"
                              n78 = call "PixelReg ProgramFromFile 2nPas.vi"("connection ID"=w400, "ACQ PxReg folder"=w393, "EQ folder path"=w394, "PixelReg (hex)"=w395, "All ID list"=w389, "Layer ID list"=w390, "Chip ID list"=w391, "error in (no error)"=w399, "PA gain"=w388, "Itest parameter"=w387, "TP EN"=w386) -> ("connection ID out"=w398:refnum<k5>, "done message"=w392:string, "All checks OK"=w396:bool, "error out (no error)"=w397:errorcluster)  [unwired: 1 out]
                              n79 = call "CloseEthConnection.vi"("error in (no error)"=w397, "connection ID"=w398) -> ("error out"=w401:errorcluster)  [unwired: 9 in]
                            }
                          }
                          n80 = case shown="True" w350 {
                            tunnel: [w367 w383] -> w343
                            tunnel: w352 -> [_ w382]
                            tunnel: w351 -> [w367 w381]
                            tunnel: [w366 w378] -> w335
                            tunnel: w342 -> [_ w377]
                            tunnel: w341 -> [_ w376]
                            tunnel: w340 -> [_ w375]
                            tunnel: [_ w374] -> w333
                            tunnel: w348 -> [_ w371]
                            tunnel: w347 -> [_ w372]
                            tunnel: w346 -> [_ w373]
                            tunnel: w349 -> [w366 _]
                            tunnel: w336 -> [_ w370]
                            tunnel: "Itest parameter" -> [_ w369]
                            tunnel: w329 -> [_ w368]
                            frame False {
                              # "Hardware 2 not enabled"
                            }
                            frame True {
                              # "Hardware 2 enabled"
                              n81 = call "PixelReg ProgramFromFile 2nPas.vi"("connection ID"=w382, "ACQ PxReg folder"=w375, "EQ folder path"=w376, "PixelReg (hex)"=w377, "All ID list"=w371, "Layer ID list"=w372, "Chip ID list"=w373, "error in (no error)"=w381, "PA gain"=w370, "Itest parameter"=w369, "TP EN"=w368) -> ("connection ID out"=w380:refnum<k5>, "done message"=w374:string, "All checks OK"=w378:bool, "error out (no error)"=w379:errorcluster)  [unwired: 1 out]
                              n82 = call "CloseEthConnection.vi"("error in (no error)"=w379, "connection ID"=w380) -> ("error out"=w383:errorcluster)  [unwired: 9 in]
                            }
                          }
                          n83 = Merge Errors(w344, w343) -> (w345:errorcluster)
                          n84 = call <vilib>:"Simple Error Handler.vi"("error in (no error)"=w345) -> ()  [unwired: 4 in, 5 out]
                          n85 = Unbundle By Name(w345) -> ("status"=w360:bool)
                          n86 = Concatenate Strings "Concatenate Strings"(w334, w339, w338, w338, w337, w333) -> (w363:string)
                          n87 = Compound Arithmetic op=AND(invert w360, w357, w335) -> (w362:bool)
                          n88 = property on="Error tick" class="Bool (strict)"(reference=w361, "Value"=w360) -> ()  [unwired: 1 in, 2 out]
                          n89 = case shown="True" w362 {
                            tunnel: w363 -> [_ w411]
                            frame False {
                              # "error"
                            }
                            frame True {
                              # "OK x2"
                              n90 = call "MessageTimeOk.vi"("time (ms)"=5200, "missage"=w411) -> ()  [unwired: 4 in]
                            }
                          }
                        }
                      }
                    }
                  }
                }
                frame #1 {
                  w414 = u32 0 ("Value")
                  # "Mostra quina EQualització carrega"
                  # "Llegeix HV final value from EQ loaded"
                  # "Inicialitza variables 'actual time'"
                  # "1) Inicialitzacions a la Adquisició. Ask for comments"
                  n91 = flat-sequence {
                    tunnel: w427 -> [w440]
                    tunnel: [w439] -> w423
                    tunnel: [w438] -> w421
                    tunnel: w420 -> [w438]
                    tunnel: [w444] -> w425
                    tunnel: [w443] -> w424
                    tunnel: w423 -> [w443]
                    tunnel: w421 -> [w442]
                    tunnel: [w447] -> w422
                    tunnel: w425 -> [w447]
                    tunnel: w424 -> [w446]
                    frame #0 {
                      n92 = property on="Operation text" class="Str"(reference=w440, "Value"="Pixel sweep acquisition...\nWrite comments for file.") -> (reference out=w439:refnum<vi>)  [unwired: 1 in, 1 out]
                    }
                    frame #1 {
                      # "ask for comments"
                      n93 = call "Acq_askComents.vi"("Folder path"=w442) -> ("Complete file path"=w444:path)  [unwired: 4 in]
                    }
                    frame #2 {
                      n94 = property on="Operation text" class="Str"(reference=w446, "Value"="Pixel sweep acquisition...") -> ()  [unwired: 1 in, 2 out]
                    }
                  }
                  n95 = property on="etapa2 Actual time" class="DigNum (strict)"(reference=w437, "Value"=w414) -> ()  [unwired: 1 in, 2 out]
                  n96 = property on="etapa5 Actual time" class="DigNum (strict)"(reference=w435, "Value"=w414) -> ()  [unwired: 1 in, 2 out]
                  n97 = property on="Events fets" class="DigNum (strict)"(reference=w415, "Value"=w414) -> ()  [unwired: 1 in, 2 out]
                  n98 = property on="Events fets A" class="DigNum (strict)"(reference=w413, "Value"=w414) -> ()  [unwired: 1 in, 2 out]
                  n99 = property on="Events fets B" class="DigNum (strict)"(reference=w412, "Value"=w414) -> ()  [unwired: 1 in, 2 out]
                  n100 = property on="etapa3 Actual time" class="DigNum (strict)"(reference=w436, "Value"=w414) -> ()  [unwired: 1 in, 2 out]
                  n101 = property on="HV parameters" class="Clust (strict)"(reference=w434) -> (reference out=w431:refnum<vi>, "Value"=w433:T5)  [unwired: 1 in, 1 out]
                  n102 = property on="Stop ACQ button" class="Bool (strict)"(reference=w419, "Value"=FALSE, "DisabledEnum"=T4."Enabled" ("Disabled"), "Visible"=TRUE) -> ()  [unwired: 1 in, 2 out]
                  n103 = in-place {
                    in-place-border: w426 -> [w448]
                    n104 = in-place-cluster #2(w433) -> ()  [unwired: 1 out]
                    n105 = in-place-cluster #2("Final value"=w448) -> (w432:T5)
                  }
                  n106 = String To Path(string=w428) -> (path=w429:path)
                  n107 = property class="Path"(reference="EQ folder path Refnum", "Value"=w429) -> ()  [unwired: 1 in, 2 out]
                  n108 = property on="HV parameters" class="Clust (strict)"(reference=w431, "Value"=w432) -> ()  [unwired: 1 in, 2 out]
                }
                frame #2 {
                  w456 = u32 0  # Comptador events per file
                  w457 = u32 1  # first file sufix num.
                  # "HV steps"
                  # "2) ADQUISICIÓ"
                  n109 = Reshape Array "Reshape Array"(w454, 5 ("dimension size"), 20 ("dimension size")) -> (w451:u8[][])
                  n110 = for {
                    tunnel: w479 -> [w510]
                    tunnel: w478 -> [w509]
                    tunnel: w477 -> [w508]
                    tunnel: w476 -> [w507]
                    tunnel: w475 -> [w506]
                    tunnel: w474 -> [w505]
                    tunnel: w473 -> [w504]
                    tunnel: w472 -> [w503]
                    tunnel: w471 -> [w502]
                    tunnel: w470 -> [w501]
                    tunnel: w469 -> [w500]
                    tunnel: w468 -> [w499]
                    tunnel: w467 -> [w498]
                    tunnel: w460 -> [w497]
                    tunnel: w466 -> [w496]
                    tunnel: w465 -> [w495]
                    tunnel: [w482] -> w450 mode=indexing
                    tunnel: w464 -> [w494]
                    tunnel: w463 -> [w493]
                    tunnel: w462 -> [w492]
                    tunnel: w461 -> [w491]
                    tunnel: w459 -> [w490]
                    tunnel: w458 -> [w489]
                    shift-right: [w480] -> _
                    shift-left: w457 -> [w488]
                    shift-right: [w481] -> _
                    shift-left: w456 -> [w487]
                    tunnel: w455 -> [w486]
                    tunnel: w451 -> [w485] mode=indexing
                    stop <- w484 stop-if-true
                    n111 = stacked-sequence {
                      tunnel: w510 -> [_ _ w568 _ _ _ _]
                      tunnel: w509 -> [_ _ w570 _ _ _ _]
                      tunnel: w508 -> [w514 _ w569 _ _ _ _]
                      tunnel: w507 -> [_ _ _ w631 _ _ _]
                      tunnel: w506 -> [w513 _ _ w630 _ _ _]
                      tunnel: w505 -> [_ _ _ _ _ w848 _]
                      tunnel: w504 -> [_ _ _ _ _ w849 _]
                      tunnel: w503 -> [w512 _ _ _ _ w847 _]
                      tunnel: w502 -> [_ w526 _ _ w806 _ _]
                      tunnel: w501 -> [_ w519 _ _ w805 _ _]
                      tunnel: w500 -> [_ w522 _ w633 w804 _ _]
                      tunnel: w499 -> [_ w517 _ _ w803 _ _]
                      tunnel: w498 -> [_ w527 w567 w627 w798 w846 w892]
                      tunnel: w497 -> [_ w524 w566 _ w800 w845 _]
                      tunnel: w496 -> [_ _ _ w635 _ _ _]
                      tunnel: w495 -> [_ _ _ w634 _ _ _]
                      tunnel: [_ _ _ w632 _ _ _] -> w483
                      tunnel: [_ _ _ _ _ _ w891] -> w484
                      tunnel: w494 -> [_ _ _ w628 _ _ _]
                      tunnel: w493 -> [_ w516 w564 _ w799 w843 _]
                      tunnel: w492 -> [_ _ w562 _ _ w841 _]
                      tunnel: w491 -> [_ _ _ w626 w796 _ _]
                      tunnel: w485 -> [_ _ _ w625 _ _ _]
                      tunnel: w490 -> [_ _ _ w623 _ _ _]
                      tunnel: w489 -> [_ _ _ w624 _ _ _]
                      tunnel: w488 -> [_ _ _ w620 _ _ _]
                      tunnel: w487 -> [_ _ _ w621 _ _ _]
                      tunnel: w486 -> [_ _ _ w622 _ _ _]
                      tunnel: [_ _ _ w619 _ _ _] -> w481
                      tunnel: [_ _ _ w618 _ _ _] -> w480
                      frame #0 {
                        w511 = u8 0 ("ACQ-e2 barra")
                        # "Inicialitzacions a la iteració"
                        n112 = property on="etapa2 barra" class="Slide (strict)"(reference=w514, "Value"=w511) -> ()  [unwired: 1 in, 2 out]
                        n113 = property on="etapa3 barra" class="Slide (strict)"(reference=w513, "Value"=w511) -> ()  [unwired: 1 in, 2 out]
                        n114 = property on="etapa5 barra" class="Slide (strict)"(reference=w512, "Value"=w511) -> ()  [unwired: 1 in, 2 out]
                      }
                      frame #1 {
                        # "Etapa 1:  rampa pujada HV"
                        n115 = flat-sequence {
                          tunnel: w527 -> [w528]
                          tunnel: w526 -> [w533]
                          tunnel: [w536] -> w525
                          tunnel: w524 -> [w535]
                          tunnel: [w534] -> w523
                          tunnel: w522 -> [w534]
                          tunnel: [w533] -> w521
                          tunnel: [w532] -> w520
                          tunnel: w519 -> [w532]
                          tunnel: [w531] -> w518
                          tunnel: w517 -> [w531]
                          tunnel: w516 -> [w529]
                          tunnel: [w528] -> w515
                          frame #0 {
                            # "Desactiva busy per permetre\nmesura de temperatura\ndurant rampa HV i temps H"
                            n116 = property on="HV level" class="Slide (strict)"(reference=w533) -> ("Value"=w539:dbl)  [unwired: 1 in, 2 out]
                            n117 = property on="Stop ACQ" class="Bool (strict)"(reference=w528) -> ("Value"=w537:bool)  [unwired: 1 in, 2 out]
                            n118 = property on="busy = F" class="Bool (strict)"(reference=w529, "Value"=FALSE) -> ()  [unwired: 1 in, 2 out]
                            n119 = Not Equal To 0?(x=w539) -> (x != 0?=w538:bool)
                            n120 = Compound Arithmetic op=OR "OR"(w538, w537, invert w535) -> (w536:bool)
                          }
                        }
                        n121 = case shown="False" w525 {
                          tunnel: w520 -> [w547 _]
                          tunnel: w521 -> [w544 _]
                          tunnel: w523 -> [w543 _]
                          tunnel: w518 -> [w541 _]
                          tunnel: w515 -> [w540 _]
                          frame False {
                            n122 = flat-sequence {
                              tunnel: [w556] -> w550
                              tunnel: w547 -> [w561]
                              tunnel: [w559] -> w546
                              tunnel: [w558] -> w545
                              tunnel: w541 -> [w555]
                              frame #0 {
                                n123 = property on="HV parameters" class="Clust (strict)"(reference=w555) -> ("Value"=w556:T5)  [unwired: 1 in, 2 out]
                                n124 = property on="HV string" class="Str"(reference=w561, "Value"="HV ramping" ("HV String"), "Text.FontColor"=u32 15365376) -> (reference out=w559:refnum<vi>, error out=w558:errorcluster)  [unwired: 1 in]
                              }
                            }
                            n125 = call "HV_drive.vi"("Stop subVI Refnum"=w540, "HV level Refnum"=w544, "HV parameters"=w550) -> ("error out"=w549:errorcluster, "HV level (last value)"=w548:dbl)  [unwired: 1 in]
                            n126 = flat-sequence {
                              tunnel: w548 -> [_]
                              tunnel: w546 -> [w553]
                              tunnel: w545 -> [w552]
                              frame #0 {
                                n127 = property on="HV string" class="Str"(reference=w553, error in=w552, "Value"="HV presence!" ("HV String"), "Text.FontColor"=u32 16711680) -> ()  [unwired: 2 out]
                              }
                            }
                            n128 = Unbundle By Name(w549) -> ("status"=w542:bool)
                            n129 = call <vilib>:"Simple Error Handler.vi"("error in (no error)"=w549) -> ()  [unwired: 4 in, 5 out]
                            n130 = property on="Error tick" class="Bool (strict)"(reference=w543, "Value"=w542) -> ()  [unwired: 1 in, 2 out]
                          }
                          frame True {
                            # "executant aturada\no hi ha HV manual\no HV not enabled"
                          }
                        }
                      }
                      frame #2 {
                        # "Etapa 2:  temps inicial a HV_H"
                        n131 = flat-sequence {
                          tunnel: w570 -> [w577]
                          tunnel: w569 -> [w576]
                          tunnel: w568 -> [w575]
                          tunnel: w567 -> [w574]
                          tunnel: w566 -> [w573]
                          tunnel: [w572] -> w565
                          tunnel: w564 -> [w572]
                          tunnel: [w571] -> w563
                          tunnel: w562 -> [w571]
                          tunnel: w565 -> [w608]
                          tunnel: w563 -> [w607]
                          frame #0 {
                            n132 = case shown="True" w573 {
                              tunnel: w577 -> [_ w583]
                              tunnel: w576 -> [_ w581]
                              tunnel: w575 -> [_ w580]
                              tunnel: w574 -> [_ w579]
                              frame False {
                              }
                              frame True {
                                n133 = property on="etapa2 Actual time" class="DigNum (strict)"(reference=w583, "Value"=u32 0 ("ACQ-e2 Actual time")) -> (reference out=w582:refnum<vi>)  [unwired: 1 in, 1 out]
                                n134 = Tick Count (ms)() -> (millisecond timer value=w584:u32)
                                n135 = while {
                                tunnel: w584 -> [w603]
                                tunnel: w582 -> [w593]
                                tunnel: w580 -> [w592]
                                tunnel: w581 -> [w590]
                                tunnel: w579 -> [w586]
                                stop <- w588 stop-if-true
                                n136 = property on="etapa2 Waiting time" class="DigNum (strict)"(reference=w592) -> ("Value"=w591:u32)  [unwired: 1 in, 2 out]
                                n137 = Tick Count (ms)() -> (millisecond timer value=w604:u32)
                                n138 = property on="Stop ACQ" class="Bool (strict)"(reference=w586) -> ("Value"=w585:bool)  [unwired: 1 in, 2 out]
                                n139 = Subtract(x=w604, y=w603) -> (x-y=w602:u32)
                                n140 = Quotient & Remainder(x=w602, y=u32 1000) -> (floor(x/y)=w594:u32)  [unwired: 1 out]
                                n141 = Greater Or Equal?(x=w594, y=w591) -> (x >= y?=w587:bool)
                                n142 = To Double Precision Float(number=w594) -> (double precision float=w595:dbl)
                                n143 = To Double Precision Float(number=w591) -> (double precision float=w596:dbl)
                                n144 = property on="etapa2 Actual time" class="DigNum (strict)"(reference=w593, "Value"=w594) -> ()  [unwired: 1 in, 2 out]
                                n145 = Divide(x=w595, y=w596) -> (x/y=w599:dbl)
                                n146 = Or(x=w587, y=w585) -> (x .or. y?=w588:bool)
                                n147 = Multiply(x=w599, y=100.0) -> (x*y=w597:dbl)
                                n148 = To Unsigned Byte Integer(number=w597) -> (unsigned 8bit integer=w589:u8)
                                n149 = property on="etapa2 barra" class="Slide (strict)"(reference=w590, "Value"=w589) -> ()  [unwired: 1 in, 2 out]
                                n150 = Wait Until Next ms Multiple(millisecond multiple=u32 100) -> ()  [unwired: 1 out]
                                }
                              }
                            }
                          }
                          frame #1 {
                            # "Reactiva busy per procedir a l'adquisició"
                            n151 = flat-sequence {
                              tunnel: w608 -> [w613]
                              tunnel: w607 -> [w611]
                              tunnel: [w611] -> w609
                              tunnel: [w610] -> w605
                              tunnel: w609 -> [w615]
                              tunnel: [w614] -> w606
                              tunnel: w605 -> [w614]
                              tunnel: w606 -> [w616]
                              frame #0 {
                                n152 = property on="busy = T" class="Bool (strict)"(reference=w613, "Value"=TRUE) -> (reference out=w610:refnum<vi>)  [unwired: 1 in, 1 out]
                              }
                              frame #1 {
                                n153 = Wait (ms)(milliseconds to wait=w615) -> ()  [unwired: 1 out]
                              }
                              frame #2 {
                                n154 = property on="busy = T" class="Bool (strict)"(reference=w616, "Value"=TRUE) -> ()  [unwired: 1 in, 2 out]
                              }
                            }
                          }
                        }
                      }
                      frame #3 {
                        # "Etapa 3:  adquisició Pixel sweep"
                        n155 = property on="Stop ACQ button" class="Bool (strict)"(reference=w627) -> ("Value"=w629:bool)  [unwired: 1 in, 2 out]
                        n156 = case shown="False" w629 {
                          tunnel: w635 -> [w646 _]
                          tunnel: w634 -> [w653 _]
                          tunnel: w633 -> [w656 _]
                          tunnel: w627 -> [w655 _]
                          tunnel: [w647 _] -> w632
                          tunnel: w631 -> [w649 _]
                          tunnel: w630 -> [w650 _]
                          tunnel: w628 -> [w648 _]
                          tunnel: w626 -> [w645 _]
                          tunnel: w625 -> [w643 _]
                          tunnel: w624 -> [w642 _]
                          tunnel: w623 -> [w641 _]
                          tunnel: w622 -> [w640 _]
                          tunnel: w621 -> [w639 w795]
                          tunnel: w620 -> [w638 w794]
                          tunnel: [w637 w795] -> w619
                          tunnel: [w636 w794] -> w618
                          frame False {
                            # "si no hi ha Stop ordenat, adquireix"
                            n157 = local read "Addresses Cluster"() -> (w654:T1)
                            n158 = Array Size(array=w643) -> (size(s)=w644:i32)
                            n159 = in-place "Conversion of DTP: ms to comptes" {
                              n160 = in-place-cluster #3("ACQ Parameters (cluster)") -> ("DTP period"=w788:u32)
                              n161 = To Double Precision Float(number=w788) -> (double precision float=w789:dbl)
                              n162 = Divide(x=w789, y=2.5e-05) -> (x/y=w792:dbl)
                              n163 = Decrement(x=w792) -> (x-1=w791:dbl)
                              n164 = To Unsigned Long Integer(number=w791) -> (unsigned 32bit integer=w790:u32)
                              n165 = in-place-cluster #3("DTP period"=w790) -> (w661:T2)
                            }
                            n166 = property class="DigNum (strict)"(reference="Events to acquire Refnum") -> ("Value"=w657:u32)  [unwired: 1 in, 2 out]
                            n167 = Cluster To Array(cluster=w661) -> (array=w651:u32[])
                            n168 = Bundle(TRUE, "Value"=w657) -> (w652:cluster{bool, "Value":u32})  [unwired: 1 in]
                            n169 = for {
                              tunnel: w656 -> [w685]
                              tunnel: w655 -> [w674]
                              tunnel: w654 -> [w684]
                              tunnel: w653 -> [w683]
                              tunnel: w652 -> [w682]
                              tunnel: w651 -> [w681]
                              tunnel: w650 -> [w680]
                              tunnel: w649 -> [w679]
                              tunnel: w648 -> [w678]
                              tunnel: [w677] -> w647 mode=indexing
                              tunnel: w646 -> [w676]
                              tunnel: w645 -> [w675]
                              tunnel: w643 -> [w671] mode=indexing
                              tunnel: w644 -> [w669]
                              tunnel: w642 -> [w668]
                              tunnel: w641 -> [w667]
                              tunnel: w640 -> [w666]
                              shift-right: [w663] -> w637
                              shift-left: w639 -> [w665]
                              shift-right: [w662] -> w636
                              shift-left: w638 -> [w664]
                              i -> [w670]
                              stop <- w673 stop-if-true
                              n170 = property on="Stop ACQ button" class="Bool (strict)"(reference=w674) -> ("Value"=w673:bool)  [unwired: 1 in, 2 out]
                              n171 = call "GlobalRegEd px_triggerEN.vi"("Pixel number"=w671, "Global Reg (default)"=w666) -> ("Global Regster (U32)"=w672:u32[])  [unwired: 3 in]
                              n172 = stacked-sequence {
                                tunnel: w685 -> [_ w702 w756 _]
                                tunnel: w674 -> [_ _ w755 _]
                                tunnel: w684 -> [_ w712 w754 _]
                                tunnel: w683 -> [_ _ w751 w783]
                                tunnel: w682 -> [_ _ w766 _]
                                tunnel: w681 -> [_ _ w765 _]
                                tunnel: w680 -> [_ _ w764 _]
                                tunnel: w679 -> [_ _ w763 _]
                                tunnel: w676 -> [_ _ w762 _]
                                tunnel: w678 -> [w689 _ w761 _]
                                tunnel: [_ _ w757 _] -> w677
                                tunnel: w672 -> [_ w706 _ _]
                                tunnel: w675 -> [w696 _ _ _]
                                tunnel: w671 -> [w691 _ _ _]
                                tunnel: w670 -> [w694 _ _ _]
                                tunnel: w669 -> [w692 _ _ _]
                                tunnel: w668 -> [w686 _ w752 _]
                                tunnel: w667 -> [w687 _ w753 _]
                                tunnel: w665 -> [_ _ _ w786]
                                tunnel: w664 -> [_ _ _ w787]
                                tunnel: [_ _ _ w784] -> w663
                                tunnel: [_ _ _ w785] -> w662
                                frame #0 {
                                w688 = u32 0 ("Value")
                                # "operation text: <px>"
                                n173 = Increment(x=w694) -> (x+1=w693:i32)
                                n174 = property on="Events fets (per pixel)" class="DigNum (strict)"(reference=w689, "Value"=w688) -> ()  [unwired: 1 in, 2 out]
                                n175 = property on="Events fets A" class="DigNum (strict)"(reference=w687, "Value"=w688) -> ()  [unwired: 1 in, 2 out]
                                n176 = property on="Events fets B" class="DigNum (strict)"(reference=w686, "Value"=w688) -> ()  [unwired: 1 in, 2 out]
                                n177 = Format Into String "Format Into String"(format string="Pixel sweep acquisition...\n(%d/%d) Central px: %d", w693, w692, w691) -> (resulting string=w690:string)  [unwired: 2 in, 1 out]
                                n178 = property on="operation text" class="Str"(reference=w696, "Value"=w690) -> ()  [unwired: 1 in, 2 out]
                                }
                                frame #1 {
                                w707 = u32 65535  # LayerID & ChipID
                                # "0) Program Glogal Reg <px>"
                                n179 = Unbundle By Name(w712) -> ("ENA1"=w708:bool, "IP address 1"=w709:string, "ENA2"=w710:bool, "IP address 2"=w711:string)
                                n180 = case shown="True" w708 {
                                tunnel: w707 -> [_ w742]
                                tunnel: [_ w745] -> w698
                                tunnel: [w737 w744] -> w700
                                tunnel: w706 -> [_ w743]
                                tunnel: w709 -> [_ w741]
                                tunnel: w710 -> [w737 _]
                                tunnel: [_ w738] -> w704
                                frame False {
                                # "Hardware 1 not enabled"
                                }
                                frame True {
                                # "Hardware 1 enabled"
                                n181 = call "OpenEthConnection.vi"("Port"=u16 80, "IP address"=w741) -> ("error out"=w749:errorcluster, "connection ID out"=w750:refnum<k5>)  [unwired: 7 in, 1 out]
                                n182 = call "ProgramGlobalReg.vi"("Global Reg"=w743, "error in (no error)"=w749, "ChipID"=w742, "LayerID"=w742, "connection ID"=w750) -> ("error out"=w739:errorcluster, "OK?"=w744:bool, "connection ID out"=w740:refnum<k5>, "Program done"=w747:string[])  [unwired: 2 in, 1 out]
                                n183 = Index Array "Index Array"(array=w747, index=1) -> (element=w745:string)
                                n184 = call "CloseEthConnection.vi"("error in (no error)"=w739, "connection ID"=w740) -> ("error out"=w738:errorcluster)  [unwired: 9 in]
                                }
                                }
                                n185 = case shown="True" w710 {
                                tunnel: w707 -> [_ w728]
                                tunnel: [_ w731] -> w697
                                tunnel: [w723 w730] -> w699
                                tunnel: w706 -> [_ w729]
                                tunnel: w711 -> [_ w727]
                                tunnel: w708 -> [w723 _]
                                tunnel: [_ w724] -> w703
                                frame False {
                                # "Hardware 2 not enabled"
                                }
                                frame True {
                                # "Hardware 2 enabled"
                                n186 = call "OpenEthConnection.vi"("Port"=u16 80, "IP address"=w727) -> ("error out"=w735:errorcluster, "connection ID out"=w736:refnum<k5>)  [unwired: 7 in, 1 out]
                                n187 = call "ProgramGlobalReg.vi"("Global Reg"=w729, "error in (no error)"=w735, "ChipID"=w728, "LayerID"=w728, "connection ID"=w736) -> ("error out"=w725:errorcluster, "OK?"=w730:bool, "connection ID out"=w726:refnum<k5>, "Program done"=w733:string[])  [unwired: 2 in, 1 out]
                                n188 = Index Array "Index Array"(array=w733, index=1) -> (element=w731:string)
                                n189 = call "CloseEthConnection.vi"("error in (no error)"=w725, "connection ID"=w726) -> ("error out"=w724:errorcluster)  [unwired: 9 in]
                                }
                                }
                                n190 = Merge Errors(w704, w703) -> (w705:errorcluster)
                                n191 = call <vilib>:"Simple Error Handler.vi"("error in (no error)"=w705) -> ()  [unwired: 4 in, 5 out]
                                n192 = Unbundle By Name(w705) -> ("status"=w701:bool)
                                n193 = disable-structure shown="Disabled" {
                                disable-tunnel: w701 -> [w720 _]
                                disable-tunnel: w700 -> [w719 _]
                                disable-tunnel: w699 -> [w718 _]
                                disable-tunnel: w698 -> [w717 _]
                                disable-tunnel: w697 -> [w715 _]
                                frame Disabled {
                                w716 = "\r"
                                n194 = Concatenate Strings "Concatenate Strings"(w717, w716, w716, w715) -> (w713:string)
                                n195 = Compound Arithmetic op=AND "AND"(invert w720, w719, w718) -> (w714:bool)
                                n196 = case shown="True" w714 {
                                tunnel: w713 -> [_ w722]
                                frame False {
                                # "error"
                                }
                                frame True {
                                # "OK x1"
                                n197 = call "MessageTimeOk.vi"("time (ms)"=1000, "missage"=w722) -> ()  [unwired: 4 in]
                                }
                                }
                                }
                                frame Enabled {
                                }
                                }
                                n198 = property on="Error tick" class="Bool (strict)"(reference=w702, "Value"=w701) -> ()  [unwired: 1 in, 2 out]
                                }
                                frame #2 {
                                # "1) Acquire Pedestal <px>"
                                n199 = local read "LayerChipIDs"() -> (w770:u16[])
                                n200 = call "subop_x2_Acquisition.vi"("ACQ stop by events"=w766, "LayerChipIDs"=w770, "ACQ parameters"=w765, "events fets A Refnum"=w753, "events fets B Refnum"=w752, "Base file path"=w751, "Addresses Cluster"=w754, "Stop ACQ button Refnum"=w755, "ACQ barra Refnum"=w764, "Actual time Refnum"=w763, "Acquisition time Refnum"=w762, "Total events Refnum"=w761) -> ("ACQ WatchDog timeout"=w757:bool, "ACQ Answer 1i2"=w758:string, "error out comm"=w760:errorcluster, "error out file"=w759:errorcluster)  [unwired: 11 in, 1 out]
                                n201 = Merge Errors(w760, w759) -> (w769:errorcluster)
                                n202 = call <vilib>:"Simple Error Handler.vi"("error in (no error)"=w769) -> ()  [unwired: 4 in, 5 out]
                                n203 = Unbundle By Name(w769) -> ("status"=w768:bool)
                                n204 = property on="Error tick" class="Bool (strict)"(reference=w756, "Value"=w768) -> ()  [unwired: 1 in, 2 out]
                                n205 = Or(x=w759, y=w757) -> (x .or. y?=w767:bool)
                                n206 = case shown="False" w767 {
                                tunnel: w758 -> [w773 _]
                                frame False {
                                # "No hi ha errors file"
                                n207 = Concatenate Strings(w773, "\r", "The file have been saved.") -> (w776:string)
                                n208 = call "MessageTimeOk.vi"("time (ms)"=1000, "missage"=w776) -> ()  [unwired: 4 in]
                                }
                                frame True {
                                # "Algun error"
                                }
                                }
                                n209 = case shown="True" w757 {
                                frame False {
                                }
                                frame True {
                                n210 = call "MessageTimeOk.vi"("time (ms)"=1000, "missage"="Acquisition WatchDog timeout." ("message")) -> ()  [unwired: 4 in]
                                }
                                }
                                }
                                frame #3 {
                                # "2) Merge temp files"
                                n211 = local read "Chip ID list 1"() -> (w781:u32[])
                                n212 = local read "Chip ID list 2"() -> (w780:u32[])
                                n213 = local read "Addresses Cluster"() -> (w782:T1)
                                n214 = To Unsigned Word Integer(number=w781) -> (unsigned 16bit integer=w779:u16[])
                                n215 = To Unsigned Word Integer(number=w780) -> (unsigned 16bit integer=w778:u16[])
                                n216 = call "ACQ PostProces1.vi"("ACQ full DATA file path"=w783, "Addresses Cluster"=w782, "Chip ID list 2"=w778, "Chip ID list 1"=w779, "events per file in"=w786, "file sufix num. in"=w787) -> ("events per file out"=w784:u32, "file sufix num. out"=w785:u32)  [unwired: 2 in, 2 out]
                                }
                              }
                            }
                          }
                          frame True {
                            # "Stop ordenat"
                          }
                        }
                      }
                      frame #4 {
                        # "Tant si hi ha Stop adquisició ordenat com si no, executa rampa baixada HV"
                        # "Etapa 4:  rampa bajada HV"
                        n217 = flat-sequence {
                          tunnel: w800 -> [w810]
                          tunnel: w799 -> [w811]
                          tunnel: [w810] -> w797
                          tunnel: w796 -> [w808]
                          frame #0 {
                            # "Desactiva busy per permetre\nmesura de temperatura\ndurant rampa HV i temps L"
                            n218 = property on="busy = F" class="Bool (strict)"(reference=w811, "Value"=FALSE) -> ()  [unwired: 1 in, 2 out]
                            n219 = property on="Operation text" class="Str"(reference=w808, "Value"="Pixel sweep acquisition...") -> ()  [unwired: 1 in, 2 out]
                          }
                        }
                        n220 = property on="HV level" class="Slide (strict)"(reference=w806) -> ("Value"=w807:dbl)  [unwired: 1 in, 2 out]
                        n221 = Not Equal To 0?(x=w807) -> (x != 0?=w802:bool)
                        n222 = And(x=w802, y=w797) -> (x .and. y?=w801:bool)
                        n223 = case shown="True" w801 {
                          tunnel: w806 -> [_ w817]
                          tunnel: w805 -> [_ w816]
                          tunnel: w804 -> [_ w815]
                          tunnel: w803 -> [_ w814]
                          tunnel: w798 -> [_ w813]
                          frame False {
                            # "HV = 0,   no cal baixada"
                          }
                          frame True {
                            n224 = flat-sequence {
                              tunnel: [w834] -> w818
                              tunnel: w816 -> [w840]
                              tunnel: [w838] -> w821
                              tunnel: [w837] -> w822
                              tunnel: w814 -> [w835]
                              frame #0 {
                                n225 = property on="HV parameters" class="Clust (strict)"(reference=w835) -> ("Value"=w834:T5)  [unwired: 1 in, 2 out]
                                n226 = property on="HV string" class="Str"(reference=w840, "Value"="HV ramping" ("HV String"), "Text.FontColor"=u32 15365376) -> (reference out=w838:refnum<vi>, error out=w837:errorcluster)  [unwired: 1 in]
                              }
                            }
                            n227 = call "HV_drive.vi"("Stop subVI Refnum"=w813, "HV level Refnum"=w817, "HV parameters"=w818) -> ("error out"=w819:errorcluster, "HV level (last value)"=w820:dbl)  [unwired: 1 in]
                            n228 = flat-sequence {
                              tunnel: w820 -> [w826]
                              tunnel: w821 -> [w833]
                              tunnel: w822 -> [w832]
                              frame #0 {
                                n229 = Equal To 0?(x=w826) -> (x = 0?=w831:bool)
                                n230 = Select(t="HV off", s=w831, f="HV presence!") -> (s? t:f=w825:string)
                                n231 = Select(t=u32 42533, s=w831, f=u32 16711680) -> (s? t:f=w824:u32)
                                n232 = property on="HV string" class="Str"(reference=w833, error in=w832, "Value"=w825, "Text.FontColor"=w824) -> ()  [unwired: 2 out]
                              }
                            }
                            n233 = Unbundle By Name(w819) -> ("status"=w823:bool)
                            n234 = call <vilib>:"Simple Error Handler.vi"("error in (no error)"=w819) -> ()  [unwired: 4 in, 5 out]
                            n235 = property on="Error tick" class="Bool (strict)"(reference=w815, "Value"=w823) -> ()  [unwired: 1 in, 2 out]
                          }
                        }
                      }
                      frame #5 {
                        # "Etapa 5:  temps final a HV_L"
                        n236 = flat-sequence {
                          tunnel: w849 -> [w856]
                          tunnel: w848 -> [w855]
                          tunnel: w847 -> [w854]
                          tunnel: w846 -> [w853]
                          tunnel: w845 -> [w852]
                          tunnel: [w851] -> w844
                          tunnel: w843 -> [w851]
                          tunnel: [w850] -> w842
                          tunnel: w841 -> [w850]
                          tunnel: w844 -> [w885]
                          tunnel: w842 -> [w884]
                          frame #0 {
                            n237 = case shown="True" w852 {
                              tunnel: w856 -> [_ w863]
                              tunnel: w855 -> [_ w860]
                              tunnel: w854 -> [_ w859]
                              tunnel: w853 -> [_ w858]
                              frame False {
                              }
                              frame True {
                                n238 = property on="etapa5 Actual time" class="DigNum (strict)"(reference=w863, "Value"=u32 0 ("ACQ-e2 Actual time")) -> (reference out=w861:refnum<vi>)  [unwired: 1 in, 1 out]
                                n239 = Tick Count (ms)() -> (millisecond timer value=w862:u32)
                                n240 = while {
                                tunnel: w862 -> [w882]
                                tunnel: w861 -> [w872]
                                tunnel: w860 -> [w871]
                                tunnel: w859 -> [w869]
                                tunnel: w858 -> [w865]
                                stop <- w867 stop-if-true
                                # "et5: temps final a HV_L"
                                n241 = property on="etapa5 Waiting time" class="DigNum (strict)"(reference=w871) -> ("Value"=w870:u32)  [unwired: 1 in, 2 out]
                                n242 = Tick Count (ms)() -> (millisecond timer value=w883:u32)
                                n243 = property on="Stop ACQ" class="Bool (strict)"(reference=w865) -> ("Value"=w864:bool)  [unwired: 1 in, 2 out]
                                n244 = Subtract(x=w883, y=w882) -> (x-y=w881:u32)
                                n245 = Quotient & Remainder(x=w881, y=u32 1000) -> (floor(x/y)=w873:u32)  [unwired: 1 out]
                                n246 = Greater Or Equal?(x=w873, y=w870) -> (x >= y?=w866:bool)
                                n247 = To Double Precision Float(number=w873) -> (double precision float=w874:dbl)
                                n248 = To Double Precision Float(number=w870) -> (double precision float=w875:dbl)
                                n249 = property on="etapa5 Actual time" class="DigNum (strict)"(reference=w872, "Value"=w873) -> ()  [unwired: 1 in, 2 out]
                                n250 = Or(x=w866, y=w864) -> (x .or. y?=w867:bool)
                                n251 = Divide(x=w874, y=w875) -> (x/y=w878:dbl)
                                n252 = Multiply(x=w878, y=100.0) -> (x*y=w876:dbl)
                                n253 = To Unsigned Byte Integer(number=w876) -> (unsigned 8bit integer=w868:u8)
                                n254 = property on="etapa5 barra" class="Slide (strict)"(reference=w869, "Value"=w868) -> ()  [unwired: 1 in, 2 out]
                                n255 = Wait Until Next ms Multiple(millisecond multiple=u32 100) -> ()  [unwired: 1 out]
                                }
                              }
                            }
                          }
                          frame #1 {
                            # "Reactiva busy per seguir amb la seqüència"
                            n256 = flat-sequence {
                              tunnel: w885 -> [w889]
                              tunnel: w884 -> [w887]
                              tunnel: [w887] -> w886
                              tunnel: w886 -> [w890]
                              frame #0 {
                                n257 = property on="busy = T" class="Bool (strict)"(reference=w889, "Value"=TRUE) -> ()  [unwired: 1 in, 2 out]
                              }
                              frame #1 {
                                n258 = Wait (ms)(milliseconds to wait=w890) -> ()  [unwired: 1 out]
                              }
                            }
                          }
                        }
                      }
                      frame #6 {
                        # "aturar adquisició?"
                        n259 = disable-structure shown="Enabled" {
                          disable-tunnel: w892 -> [w894 _]
                          disable-tunnel: [w893 w895] -> w891
                          frame Enabled {
                            n260 = property on="Stop ACQ" class="Bool (strict)"(reference=w894) -> ("Value"=w893:bool)  [unwired: 1 in, 2 out]
                          }
                          frame Disabled {
                            w895 = TRUE  # only one HV run
                          }
                        }
                      }
                    }
                    n261 = And Array Elements(Boolean array=w483) -> (logical AND=w482:bool)
                  }
                  n262 = And Array Elements(Boolean array=w450) -> (logical AND=w449:bool)
                }
                frame #3 {
                  # "3) Finalització a l'adquisició. Restaura Global Registers."
                  n263 = flat-sequence {
                    tunnel: w901 -> [w904]
                    tunnel: [w904] -> w900
                    tunnel: w899 -> [w903]
                    tunnel: w900 -> [w906]
                    tunnel: w896 -> [w905]
                    tunnel: w898 -> [w955]
                    tunnel: w897 -> [w954]
                    frame #0 {
                      n264 = property on="operation text" class="Str"(reference=w903, "Value"="Pixel sweep acquisition...\nRestoring Global Regs.") -> ()  [unwired: 1 in, 2 out]
                    }
                    frame #1 {
                      w911 = "\r"
                      w919 = u32 65535  # LayerID & ChipID
                      # "Restaura Global Registers."
                      n265 = local read "Addresses Cluster"() -> (w907:T1)
                      n266 = Unbundle By Name(w907) -> ("ENA1"=w920:bool, "IP address 1"=w921:string, "ENA2"=w922:bool, "IP address 2"=w923:string)
                      n267 = case shown="True" w920 {
                        tunnel: w919 -> [_ w945]
                        tunnel: [_ w948] -> w912
                        tunnel: [w940 w947] -> w914
                        tunnel: w905 -> [_ w946]
                        tunnel: w921 -> [_ w944]
                        tunnel: w922 -> [w940 _]
                        tunnel: [_ w941] -> w917
                        frame False {
                          # "Hardware 1 not enabled"
                        }
                        frame True {
                          # "Hardware 1 enabled"
                          n268 = call "OpenEthConnection.vi"("Port"=u16 80, "IP address"=w944) -> ("error out"=w952:errorcluster, "connection ID out"=w953:refnum<k5>)  [unwired: 7 in, 1 out]
                          n269 = call "ProgramGlobalReg.vi"("Global Reg"=w946, "error in (no error)"=w952, "ChipID"=w945, "LayerID"=w945, "connection ID"=w953) -> ("error out"=w942:errorcluster, "OK?"=w947:bool, "connection ID out"=w943:refnum<k5>, "Program done"=w950:string[])  [unwired: 2 in, 1 out]
                          n270 = Index Array "Index Array"(array=w950, index=1) -> (element=w948:string)
                          n271 = call "CloseEthConnection.vi"("error in (no error)"=w942, "connection ID"=w943) -> ("error out"=w941:errorcluster)  [unwired: 9 in]
                        }
                      }
                      n272 = case shown="True" w922 {
                        tunnel: w919 -> [_ w931]
                        tunnel: [_ w934] -> w910
                        tunnel: [w926 w933] -> w913
                        tunnel: w905 -> [_ w932]
                        tunnel: w923 -> [_ w930]
                        tunnel: w920 -> [w926 _]
                        tunnel: [_ w927] -> w916
                        frame False {
                          # "Hardware 2 not enabled"
                        }
                        frame True {
                          # "Hardware 2 enabled"
                          n273 = call "OpenEthConnection.vi"("Port"=u16 80, "IP address"=w930) -> ("error out"=w938:errorcluster, "connection ID out"=w939:refnum<k5>)  [unwired: 7 in, 1 out]
                          n274 = call "ProgramGlobalReg.vi"("Global Reg"=w932, "error in (no error)"=w938, "ChipID"=w931, "LayerID"=w931, "connection ID"=w939) -> ("error out"=w928:errorcluster, "OK?"=w933:bool, "connection ID out"=w929:refnum<k5>, "Program done"=w936:string[])  [unwired: 2 in, 1 out]
                          n275 = Index Array "Index Array"(array=w936, index=1) -> (element=w934:string)
                          n276 = call "CloseEthConnection.vi"("error in (no error)"=w928, "connection ID"=w929) -> ("error out"=w927:errorcluster)  [unwired: 9 in]
                        }
                      }
                      n277 = Merge Errors(w917, w916) -> (w918:errorcluster)
                      n278 = call <vilib>:"Simple Error Handler.vi"("error in (no error)"=w918) -> ()  [unwired: 4 in, 5 out]
                      n279 = Unbundle By Name(w918) -> ("status"=w915:bool)
                      n280 = Concatenate Strings "Concatenate Strings"(w912, w911, w911, w910) -> (w908:string)
                      n281 = Compound Arithmetic op=AND "AND"(invert w915, w914, w913) -> (w909:bool)
                      n282 = property on="Error tick" class="Bool (strict)"(reference=w906, "Value"=w915) -> ()  [unwired: 1 in, 2 out]
                      n283 = case shown="True" w909 {
                        tunnel: w908 -> [_ w925]
                        frame False {
                          # "error"
                        }
                        frame True {
                          # "OK x1"
                          n284 = call "MessageTimeOk.vi"("time (ms)"=1000, "missage"=w925) -> ()  [unwired: 4 in]
                        }
                      }
                    }
                    frame #2 {
                      w956 = FALSE ("Value")
                      # "Desactiva busy per permetre\nmesura de temperatura\ndurant ACQ data viewer."
                      n285 = property on="Stop ACQ button" class="Bool (strict)"(reference=w955, "Visible"=w956, "Value"=w956, "DisabledEnum"=T4."Enabled" ("Disabled")) -> ()  [unwired: 1 in, 2 out]
                      n286 = property on="busy = F" class="Bool (strict)"(reference=w954, "Value"=FALSE) -> ()  [unwired: 1 in, 2 out]
                    }
                  }
                }
                frame #4 {
                  # "4) Open DATA viewer"
                  n287 = local read "ACQ Parameters (cluster)"() -> (w972:T2)
                  n288 = property on="ACQ events fets" class="DigNum (strict)"(reference=w963) -> ("Value"=w974:u32)  [unwired: 1 in, 2 out]
                  n289 = property on="etapa2 Waiting time (s)" class="DigNum (strict)"(reference=w959) -> ("Value"=w971:u32)  [unwired: 1 in, 2 out]
                  n290 = property on="etapa5 Waiting time (s)" class="DigNum (strict)"(reference=w960) -> ("Value"=w970:u32)  [unwired: 1 in, 2 out]
                  n291 = property on="Acquisition time (s)" class="DigNum (strict)"(reference=w961) -> ("Value"=w969:u32)  [unwired: 1 in, 2 out]
                  n292 = local read "GbReg params"() -> (w975:u8[])
                  n293 = property on="HV parameters" class="Clust (strict)"(reference=w962) -> ("Value"=w973:T5)  [unwired: 1 in, 2 out]
                  n294 = Index Array "Index Array"(array=w975) -> (element #1=w968:u8, element #2=w967:u8)  [unwired: 2 in]
                  n295 = call "Grava_conditionsACQ.vi"("ACQ Parameters (cluster)"=w972, "HV parameters"=w973, "ACQ events fets"=w974, "EQ folder path"=w964, "ACQ folder path"=w965, "EQ loaded?"=w966, "etapa2 Waiting time (s)"=w971, "ACQ anVref low"=w968, "Acquisition time (s)"=w969, "ACQ GbTHLD"=w967, "etapa5 Waiting time (s)"=w970) -> ()  [unwired: 9 in]
                  n296 = disable-structure shown="Disabled" {
                    disable-tunnel: w979 -> [w984 _]
                    disable-tunnel: w978 -> [w983 _]
                    disable-tunnel: w977 -> [w982 _]
                    disable-tunnel: w963 -> [w981 _]
                    disable-tunnel: w976 -> [w980 _]
                    frame Disabled {
                      n297 = case shown="False" w984 {
                        tunnel: w983 -> [w992 _]
                        tunnel: w982 -> [w991 _]
                        tunnel: w981 -> [w990 _]
                        tunnel: w980 -> [w986 _]
                        frame False {
                          # "No hi ha timeout: obre DATA viewer"
                          n298 = flat-sequence {
                            tunnel: w990 -> [w998]
                            tunnel: w991 -> [w999]
                            tunnel: w992 -> [w1000]
                            tunnel: [w1000] -> w989
                            tunnel: [w999] -> w988
                            tunnel: [w998] -> w987
                            tunnel: w986 -> [w997]
                            tunnel: [w993] -> w985
                            tunnel: w989 -> [w1008]
                            tunnel: w988 -> [w1012]
                            tunnel: w987 -> [w1011]
                            tunnel: w985 -> [w1009]
                            frame #0 {
                              n299 = local read "Chip ID list 1"() -> (w995:u32[])
                              n300 = local read "Chip ID list 2"() -> (w994:u32[])
                              n301 = Build Array (concatenate) "Concatenate"(w995, w994) -> (w993:u32[])
                              n302 = property on="Operation text" class="Str"(reference=w997, "Value"="Pixel sweep acquisition...\nData viewer open") -> ()  [unwired: 1 in, 2 out]
                            }
                            frame #1 {
                              n303 = Strip Path(path=w1008) -> (stripped path=w1007:path)  [unwired: 1 out]
                              n304 = List Folder(path=w1007, pattern="*.dat") -> (filenames=w1005:string[])  [unwired: 2 in, 3 out]
                              n305 = Array Size(array=w1005) -> (size(s)=w1004:i32)
                              n306 = for {
                                N: w1004 -> [_]
                                tunnel: w1009 -> [w1026]
                                tunnel: w1008 -> [w1028]
                                shift-right: [w1030] -> _
                                shift-left: w1004 -> [w1031]
                                tunnel: [w1029] -> w1002
                                tunnel: [w1027] -> w1003
                                tunnel: [w1026] -> w1001
                                n307 = To Unsigned Long Integer(number=w1031) -> (unsigned 32bit integer=w1032:u32)
                                n308 = Decrement(x=w1031) -> (x-1=w1030:i32)
                                n309 = call "Grava_summaryACQ.vi"("sufix number"=w1032, "ChipID list"=w1026, "ACQ full DATA file path"=w1028) -> ("quants events per chip"=w1029:u32[], "suffixed file path"=w1027:path)  [unwired: 1 in]
                              }
                              n310 = property class="DigNum (strict)"(reference=w1011) -> ("Value"=w1010:u32)  [unwired: 1 in, 2 out]
                              n311 = disable-structure shown="Disabled" {
                                disable-tunnel: w1012 -> [w1018 _]
                                disable-tunnel: w1010 -> [w1017 _]
                                disable-tunnel: w1004 -> [w1016 _]
                                disable-tunnel: w1003 -> [w1015 _]
                                disable-tunnel: w1002 -> [w1014 _]
                                disable-tunnel: w1001 -> [w1013 _]
                                frame Disabled {
                                # "No obrir per falta de memòria en WinXP"
                                n312 = case shown="1" w1016 {
                                tunnel: w1018 -> [_ w1025]
                                tunnel: w1017 -> [_ w1024]
                                tunnel: w1015 -> [_ w1023]
                                tunnel: w1014 -> [_ w1021]
                                tunnel: w1013 -> [_ w1022]
                                frame Default {
                                # "Empty file path\nEmpty ChipID list"
                                # "to choose ACQ file"
                                n313 = call "ACQ_Data_viewer (Module).vi"("ACQ full DATA file path"=path "", "ChipID list"=u32[] []) -> ()  [unwired: 14 in]
                                }
                                frame 1 {
                                # "only one ACQ file"
                                n314 = call "ACQ_Data_viewer (Module).vi"("ACQ full DATA file path"=w1023, "ChipID list"=w1022, "quants events per chip"=w1021, "ID summary"=w1025, "ACQ events fets"=w1024) -> ()  [unwired: 11 in]
                                }
                                }
                                }
                                frame Enabled {
                                }
                              }
                            }
                          }
                        }
                        frame True {
                        }
                      }
                    }
                    frame Enabled {
                    }
                  }
                }
              }
            }
          }
        }
      }
    }
    frame True {
      # "connection not working"
      n315 = property on="Error tick" class="Bool (strict)"(reference=w1033, "Value"=w1034) -> ()  [unwired: 1 in, 2 out]
      n316 = One Button Dialog(message="The connection is NOT WORKING.\n\nCheck the wiring connection and the IP address.") -> ()  [unwired: 1 in, 1 out]
    }
  }
  "Folder path: acquisition reports" <- w1
